vi "UHR-Fleezers Control (fpga) - avogadro 4.vi"() -> ()   [LabVIEW 2014]
doc: "UHR-Fleezers Instrument Control Code (fpga)"
uses:
  <vilib>/Platform/TimedLoop/XDataNode/timing_clust.ctl
  <vilib>/Platform/TimedLoop/XDataNode/nitl_modes.ctl
  <vilib>/Platform/TimedLoop/XDataNode/wakeup.ctl
  <vilib>/rvi/Emulation/niFpgaGetClockAttributes.vi
  <vilib>/rvi/Emulation/niFpgaSctlEmulationGetInTimedLoop.vi
  <vilib>/rvi/Emulation/niFpgaEmulationReportErrorSimple.vi
  <vilib>/rvi/Emulation/niFpgaProcessEmulError.vi
  <vilib>/rvi/eio/common/nirviEmuTemplateMethod_errors.vi
  <vilib>/rvi/Emulation/niFpgaEmulationIsFPGAContextNoSignature.vi
  <vilib>/rvi/errors/niFpgaSetErrorForExecOnDevCompSimple.vi
  <vilib>/rvi/eio/common/nirviEmuReportErrorAndStop.vi
  <vilib>/rvi/DataTransferAndStorage/Container/Common/niFpgaContainerGetUniqueNameForEmu.vi
  <vilib>/rvi/FIFO/Fifo_Resource/nirvififoEmulationSetSize.vi
  <vilib>/rvi/FIFO/Fifo_Resource/nirviFifoEmulationQueueMgr.vi
  <instcachedir>/0/nirviFifoEmulationQueueMgr_E5CAEC123FF24DC58D834DCA3CDAA9B5.lvgen/nirviFifoEmulationQueueMgr_E5CAEC123FF24DC58D834DCA3CDAA9B5_001.vi
  <vilib>/Utility/error.llb/Clear Errors.vi
  <vilib>/rvi/FIFO/Fifo_Resource/nirvififoEmulationCreateLock.vi
  <vilib>/rvi/FIFO/Fifo_Resource/nirvififoEmulationObtainLock.vi
  <vilib>/rvi/FIFO/Fifo_Resource/nirvififoEmulationReleaseLock.vi
  <vilib>/rvi/occurrence/nirviWaitOnOccurrenceBase.vi
  <vilib>/rvi/errors/nirviReportUnexpectedCaseInternalError.vi
  <vilib>/rvi/errors/nirviReportUnexpectedCaseInternalError (U32).vi
  <vilib>/rvi/DataTransferAndStorage/Container/Common/niFpgaContainerExecOnDevCompGetState.vi
  <vilib>/rvi/FIFO/Fifo_Resource/nirvififoEmulationDetermineInputValidOut.vi
  <vilib>/rvi/interface/RandomDataEmulation/niFpgaRandomDataHandleErrors.vi
  <vilib>/rvi/Emulation/niFpgaCriticalErrorInLSC.vi
  <vilib>/rvi/Memory/Memory_Emulation/niFpgaMemoryEmulationCacheClearOnFirstRun.vi
  <vilib>/rvi/Memory/Memory_Emulation/nirvimemoryEmulationManagerCache_MakeExclusive.vi
  <vilib>/rvi/Memory/Memory_Emulation/niFpgaMemoryEmulationValidateCache.vi
  <vilib>/rvi/Memory/Memory_Emulation/nirvimemoryEmulationManagerCache_InsertValue.vi
  <vilib>/rvi/Memory/Memory_Emulation/nirvimemoryEmulationManagerCache_ReleaseExclusive.vi
  <vilib>/rvi/Memory/Memory_Emulation/nirvimemoryEmulationManagerCache_GetValue.vi
  <vilib>/rvi/Memory/Memory_Emulation/nirvimemoryEmulationManagerCache_SetValue.vi
  <vilib>/rvi/Emulation/niFpgaSctlEmulationResourceMgr.vi
  <vilib>/eio/EIONode/EIONode.xnode
  <vilib>/eio/EIOMethodNode/EIOMethodNode.xnode
  <vilib>/Platform/TimedLoop/XDataNode/XDataNode.xnode
  <vilib>/rvi/DataTransferAndStorage/Container/XNode/niFpgaContainer.xnode
  <vilib>/rvi/FIFO/Fifo_Resource/nirvififoEmulationRead.vi
  <vilib>/rvi/FIFO/Fifo_Resource/niFpgaFifoEmulationRefIn.vi
  <vilib>/rvi/interface/RandomDataEmulation/nirviRandomDataFpgaReadWriteTemplate.vi
  <vilib>/rvi/FIFO/Fifo_Resource/nirvififoEmulationWrite.vi
  <vilib>/rvi/Memory/Memory_Emulation/niFpgaMemoryEmulationRefIn.vi
  <vilib>/addons/control/pid/fpga.llb/XNode/niFpgaPID.xnode
  <vilib>/Platform/TimedLoop/XDataNode/XDNodeRunTimeDep.lvlib
panel:
  in  "BD 1 Delay (ticks)":u8
  out "lifetime (ticks)":u16
  in  "Lifetime to FIFO":bool
  in  "Tab Control":T1(tab)=enum."MCL trap control"
  in  "Set 3":bool
  in  "Set 2":bool=TRUE
  in  "Set 1":bool=TRUE
  in  "Trap Pos to FIFO":bool
  in  "N of AI1 Int Acq Sets":i16=2 min=1 max=3 step=1
  out "AI Late Counter":u8
  in  "ai count":u16=400
  in  "+ phase":bool
  in  "Phase count adjustment":i16
  out "Relative phase":i16
  in  "AI to FIFO":bool
  out "BD1 Frequency Out 1":u64
  out "BD1 Frequency Out 2":u64
  out "Trap Pos FIFO Timeout":u16
  out "Trap AI FIFO Timeout":u16
  in  "Trap FIFO Set Timeout":i32
  in  "Tab Control 2":T2(tab)
  in  "Multiple trap 3 position offset \nfile":bool
  in  "Piezo offset Y points":u64
  in  "Piezo offset X points":u64
  in  "Piezo offset Xmin":u64
  in  "Piezo Offset Ymin":u64
  in  "Piezo Offset Increment":u64
  out "BD1 amplitude 1 out":u16
  out "BD1 amplitude 2 out":u16
  in  "FB output range":cluster{"output low":i16, "output high":i16}={"output low"=0, "output high"=3000}
  in  "FB Gains":T3={"proportional gain (Kc)"=10, "integral gain (Kc*Ts/Ti)"=5, "derivative gain (Kc*Td/Ts)"=0}
  in  "RF synth green feedback max":i16=4000
  in  "RD":bool=TRUE
  in  "Swap F1 and F2":bool
  in  "Cont. Scan":bool
  in  "Abort scan":bool
  in  "Cycles per step":u64
  in  "Scan BD":bool
  in  "Number of scans":u16
  in  "Scan steps":u64
  in  "Scan freq.  increment":i64
  out "Scanning":bool
  in  "Start scan":bool
  in  "OSK Bd 1":bool
  in  "Reset Bd 1":bool
  in  "PMODE":bool=TRUE
  in  "Number Interlace Cycles":u8=2 min=1 max=3
  in  "Interlace Off Parameters":u8=1 min=1 max=3
  in  "Interlace ON/OFF":bool
  out "DIO Relative phase":i16
  in  "Phase count adjustment (DIO)":i16
  in  "+ phase (DIO)":bool
  out "DIO Late Counter":u8
  in  "DIO count 1 (ticks)":u16=400
  in  "DIO count 2 (ticks)":u16=400
  in  "DIO count 3 (ticks)":u16=400
  out "AI2 Y Sum Set 2":i16
  out "AI2 Y Sum Set 1":i16
  in  "FB Setpoint Set 1":i16 min=0 step=1
  in  "FB Reset Set 1":bool
  in  "FB On/Off Set 1":bool
  in  "FB Reset Set 2":bool
  in  "FB On/Off Set 2":bool
  in  "FB Setpoint Set 2":i16 min=0 step=1
  out "Scan I":u64
  in  "Amp switch delay":u8=5
  in  "RF synth bd controls green":bool
  in  "Phase Trap 2":fxp<+,14,14>
  in  "Phase Trap 1":fxp<+,14,14>
  in  "Phase offset method":u8
  in  "BD 2 Amplitude 1":u16
  in  "BD 1 Amplitude 1":u16
  in  "BD 2 Frequency 1":u64
  in  "BD 1 Frequency 1":u64
  in  "BD 2 Amplitude 2":u16
  in  "BD 1 Amplitude 2":u16
  in  "BD 2 Frequency 2":u64
  in  "BD 1 Frequency 2":u64
  in  "BD 2 Amplitude 3":u16
  in  "BD 1 Amplitude 3":u16
  in  "BD 2 Frequency 3":u64
  in  "BD 1 Frequency 3":u64
  in  "BD 2 Delay (Ticks)":u8 caption="Count(Ticks)"
  in  "Next trap write delay (ticks)":u8 caption="Count(Ticks)"
  out "Random phase generated":fxp<+,14,14>
  in  "RF phase reset before cycles":bool
  in  "Trap 1 osc enable":bool
  in  "N trap osc periods":i16
  in  "Trap osc period (pts)":i16
  in  "Osc traps":bool
  in  "Initiate trap osc":bool
  in  "Ready Write":bool
  in  "Data":i64
  in  "Address 2":u32
  in  "Osc trap cont.":bool
  in  "Trap 2 osc enable":bool
  out "Piezo X out":i16
  out "Piezo Y out":i16
  in  "Piezo Trap ON/Off (AO3)":i16
  in  "Piezo Trap X (AO5)":i16
  in  "Piezo Trap Y (AO4)":i16
  in  "FB Min frequency":u64
  in  "FB Max Frequency":u64
  in  "Dynamic Force FB (Ronen)":bool
  in  "Trap pos. FB Range":T4={"FB2 output low"=-1.0, "FB2 output high"=0.999969482421875}
  in  "Trap Pos. FB Gains":T5={"proportional gain (Kc)"=0.999969482421875, "integral gain (Kc*Ts/Ti)"=0.999969482421875, "derivative gain (Kc*Td/Ts)"=0.0}
  in  "B factor":fxp<+/-,32,16>
  in  "Negate Diff?":bool
  in  "Diff FB Measurement?":bool
  in  "FB Trig Integrate":u32=1
  out "TTrig?":bool
  in  "TTrig Negate Pos":bool=TRUE
  out "Trap Pos FB Int Signal":fxp<+/-,24,9> format="%.18g"
  out "Trap Pos FB Int-Norm Signal":fxp<+/-,16,1> format="%.16g"
  in  "FPGA TTrig Thresh":i64
  in  "FPGA Trap Trig":bool
  out "Trap Pos FB Action":i64
  in  "Trap Pos. FB Offset Factor":i64
  in  "Trap Pos. FB Mult Factor":i64=2
  in  "Trap Pos. FB Reset":bool
  in  "Trap Pos FB Monitor T1 or T2":bool
  in  "AI1 X Scale":u16
  in  "Trap Pos FB Int Count":u16=100
  in  "Trap Pos FB Negate Action":bool
  out "AI1 X Set 2":fxp<+/-,16,1>
  out "AI1 X Set 1":fxp<+/-,16,1>
  in  "Trap Pos. FB SP":fxp<+/-,16,1>
  in  "Force feedback":bool
  out "TTrig Sig":i64
  out "TTrig Fin Thresh":i64
  in  "ScanTrap 3 or Fl-laser":bool
  in  "1D or 2D Scan?":bool
  in  "Abort scan (MCL)":bool
  in  "MCL Scan Axis":bool
  in  "Cont. Scan (MCL)":bool
  out "Scan I (MCL)":u64
  in  "Number of scans (MCL)":u16
  out "Scanning MCL":bool
  in  "Scan steps (MCL)":u64
  in  "Cycles per step (MCL)":u64
  in  "Scan freq.  increment (MCL)":i16
  in  "Start scan (MCL)":bool
  in  "AO2 (X)":i16
  in  "AO1 (Y)":i16
  out "MCL Late Counter":u8
  in  "MCL count":u32=800
  out "MCL Relative Phase":i16
  in  "Phase count adjustment (MCL)":i16
  in  "+ phase (MCL)":bool
  in  "Lifetime events to read blue":u16=100
  in  "Lifetime read blue fifo":bool
  out "lifetime events in fifo":u16
  out "APD2 int gate":bool
  out "APD3 out state":bool
  in  "APD Gate Operating Mode":u8 max=2 step=1
  in  "Invert APD Gate":bool
  in  "APD Gate OFF Count":u16=100
  in  "APD Gate ON Count":u16=300
  out "APD 1 Gate Late Counter":u8
  out "APD 1 Gate Relative Phase":i16
  in  "Phase count adjustment (APD 1 Gate)":i16
  in  "+ phase (APD 1 Gate)":bool
  out "APD 2 Counts 0":u32
  out "APD 2 Counts 1":u32
  out "APD 1 Counts 0":u32
  out "APD 1 Counts 1":u32
  out "APD1 out state":bool
  in  "APD AO scale factor":i16=1
  in  "APD to FIFO":bool
  in  "APD Acq Rate Count":u32=20000000
  out "APD Acq Late Counter":u8
  out "APD Acq Relative Phase":i16
  in  "Phase Count Adjustment (APD Acq)":i16
  in  "+ phase (APD Acq)":bool
  in  "Phase count adjustment (APD 2 Gate)":i16
  out "APD 2 Gate Late Counter":u8
  out "APD 2 Gate Relative Phase":i16
  in  "+ phase (APD 2 Gate)":bool
  out "APD2 out state":bool
  out "APD 3 Counts 0":u32
  out "APD 3 Counts 1":u32
  out "APD 3 Gate Late Counter":u8
  in  "Phase count adjustment (APD 3 Gate)":i16
  out "APD 3 Gate Relative Phase":i16
  in  "+ phase (APD 3 Gate)":bool
  out "APD1 int gate":bool
  out "APD3 int gate":bool
  in  "Lifetime timeout APD1":u16=200
  in  "D3 2":i16
  in  "I3 2":i16=5
  in  "P3 2":i16=10
  in  "Green FB Setpoint 2":i16=250 min=0 step=1
  in  "Green FB Reset 2":bool
  in  "ALEX ON":bool
  out "ALEX green ON":bool=TRUE
  in  "ALEX green on count":i16=1
  in  "D3":i16
  in  "I3":i16=5
  in  "P3":i16=10
  in  "Green Filter Flipper":bool
  in  "Green FB Count":u16=1200
  out "Green Late Counter":u8
  out "Green FB Relative Phase":i16
  in  "Phase count adjustment (Green FB)":i16=10
  in  "+ phase (Green FB)":bool
  out "Green FB Sum":i16
  in  "Green int current ON count adj":u16=150
  in  "Current Out":u16=30000
  in  "Green FB On/Off":bool
  in  "Green FB Setpoint":i16=250 min=0 step=1
  in  "Green FB Reset":bool
  in  "Operating Mode 2":u8=2 max=2 step=1
  in  "Invert GI 2":bool
  in  "Green interlace OFF count 2":u16=900
  in  "Green interlace ON count 2":u16=300
  out "GI Late Counter 2":u8
  out "GI Relative phase 2":i16
  in  "Phase count adjustment (GI) 2":i16=20
  in  "+ phase (GI) 2":bool
  in  "Green interlace OFF count":u16=100
  out "GI Relative phase":i16
  in  "Phase count adjustment (GI)":i16
  in  "+ phase (GI)":bool
  in  "Green interlace ON count":u16=300
  out "GI Late Counter":u8
  in  "Invert GI":bool
  in  "Operating Mode":u8 max=2 step=1
  in  "ALEX red on count":i16=1
  out "ALEX red ON":bool=TRUE
  out "green FB running":bool
  in  "+ phase (RI)":bool
  out "RI Relative phase":i16
  out "RI Late Counter":u8
  in  "Red interlace ON count":u16=300
  in  "Red interlace OFF count":u16=100
  in  "Invert RI":bool
  in  "Red Laser Operating Mode":u8 max=2 step=1
  in  "Phase count adjustment (RI)":i16
  out "Red FB Intensity":i16
  in  "RI Current Out":u16=30000
  in  "Red FB On/Off":bool
  in  "D4":i16
  in  "I4":i16=5
  in  "P4":i16=10
  in  "Red FB Setpoint":i16=250 min=0 step=1
  in  "Red FB Reset":bool
  in  "RI Operating Mode 2":u8=2 max=2 step=1
  in  "Invert RI 2":bool
  in  "Phase count adjustment (BI AO)":i16=20
  in  "Blue current ON count adj (AO)":u16=150
  in  "BI Current Out":i16=30000
  in  "Blue FB On/Off":bool
  in  "D5":i16
  in  "I5":i16=5
  in  "P5":i16=10
  in  "Blue FB Setpoint":i16=250 min=0 step=1
  in  "Blue FB Reset":bool
  in  "BI Operating Mode (AO)":u8=2 max=2 step=1
  in  "Invert BI (AO)":bool
  in  "Blue OFF count (AO)":u16=900
  in  "Blue ON count (AO)":u16=300
  out "BI Late Counter (AO)":u8
  out "BI Relative phase (AO)":i16
  in  "+ phase (BI AO)":bool
  in  "Phase count adjustment (BI D)":i16
  in  "Blue Laser Operating Mode (D)":u8 max=2 step=1
  in  "Invert BI (D)":bool
  in  "Blue interlace OFF count (D)":u16=100
  in  "Blue interlace ON count (D)":u16=300
  out "Blue Late Counter (D)":u8
  out "BI Relative phase (D)":i16
  in  "+ phase (BI D)":bool
  out "Blue Intensity":i16
  # "Raster Scan AOD"
  # "1 (X)"
  # "2 (Y)"
  # "IR Intensity Feedback (RF BD 1)"
  # "FB Gains Set 1"
  # "FB output range 1"
  # "IR Intensity Feedback (RF BD 2) -\nonly when using BD 2 for green laser AOM (not trap Y)"
  # "Keep below 4096 (12 bits) to stay within range of RF board. Going over doesn't saturate, it truncates higher bits."
  # "RF phase offset control"
  # "Methods are:\n0 - Default, do nothing at all (no phase offset writes)\n1 - Manual phase adjustment\n2 - Cycle the phase adjustment using the input phase numbers as increment values for each cycle"
  # "False is usual, True is external loop method"
  # "Parameters if using the external RF switching loop"
  # "Parameters if using the usual internal RF switching method"
  # "FB Triggering Excitation Laser"
  # "Trap Pos. FB Gains"
  # "Trap Pos. FB Range"
  # "AO1 (Y)"
  # "2D"
  # "Trap 3"
  # "1D"
  # "AO2 (X)"
  # "Fl Laser"
  # "APD AO for aligning"
  # "Detection Loop"
  # "Green fluorescent laser digital gate interlacing loop"
  # "0 Forced ON\n1 Forced OFF\n2 Interlacing"
  # "ALEX settings:"
  # "Controls for usual IA ME controls green AOM"
  # "Controls for RF synth board controls green AOM"
  # "Green FB Gains"
  # "Red fluorescent laser digital gate interlacing loop"
  # "Detection Loop"
  # "0 Forced ON\n1 Forced OFF\n2 Interlacing"
  # "Analog/FB Control Loop\n(Disabled)"
  # "Digital Control Loop"
  # "Blue laser intensity reading"
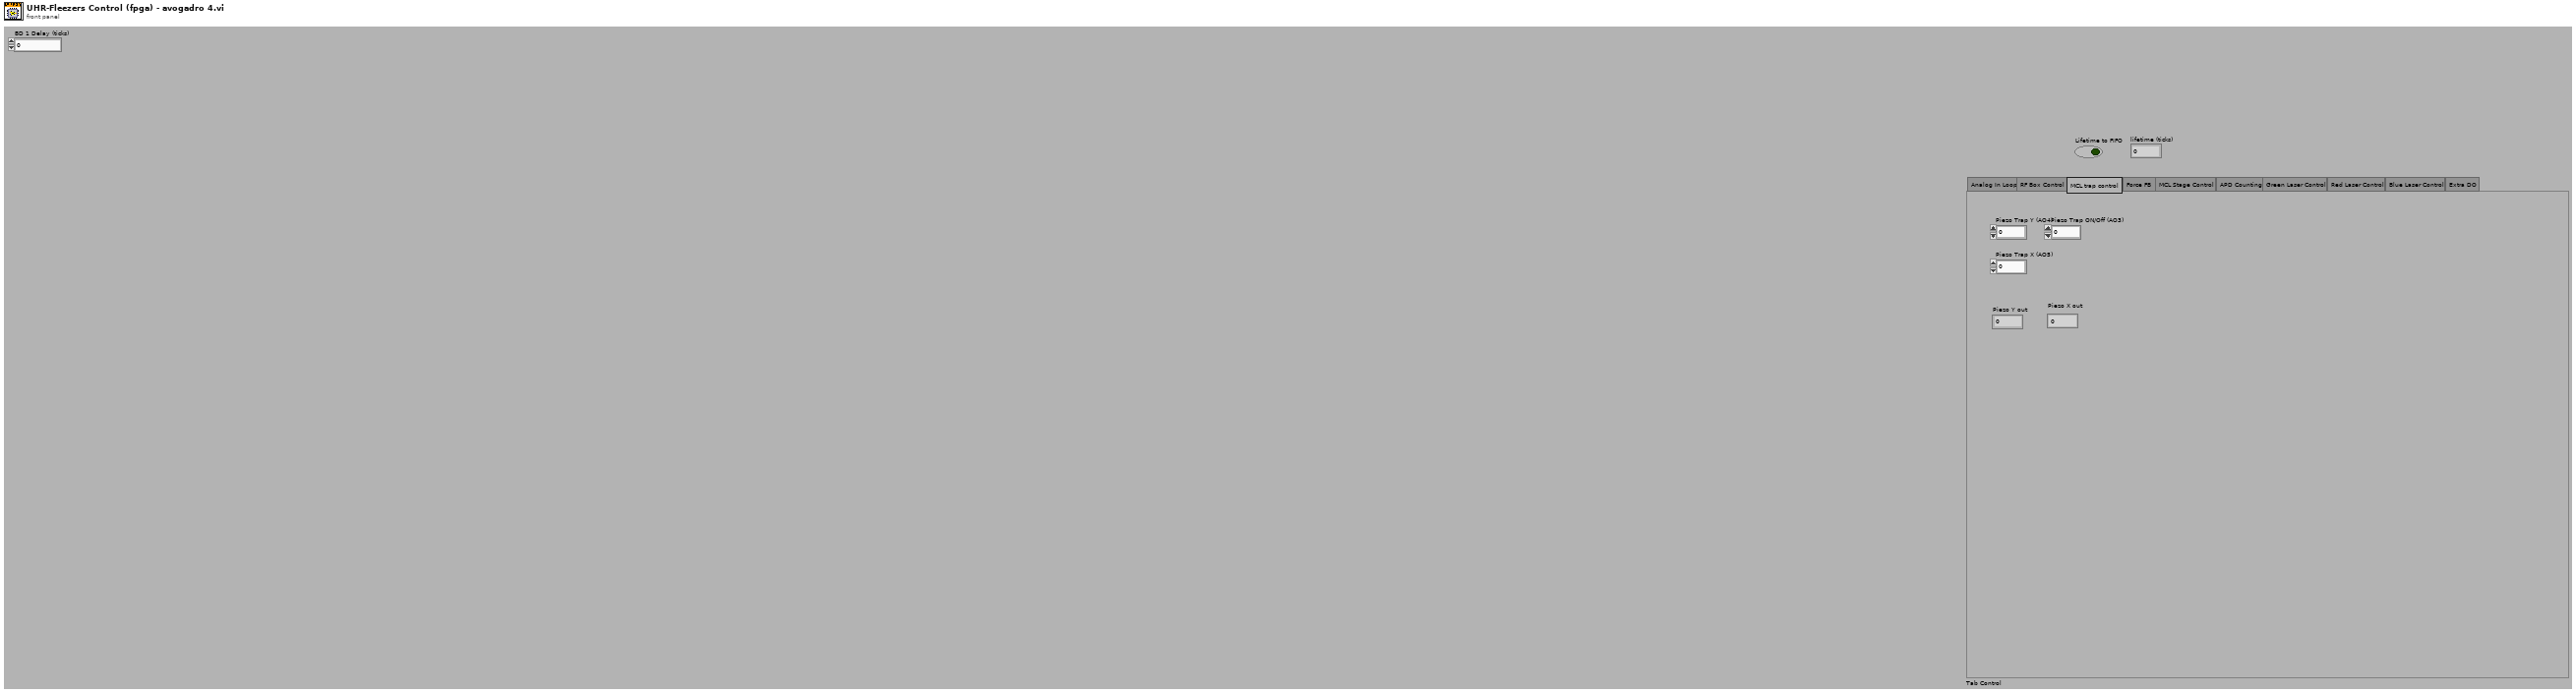
[diagram p1: front panel]
types:
  T1 = enum32{"Analog In Loop", "RF Box Control", "MCL trap control", "Force FB", "MCL Stage Control", "APD Counting", "Green Laser Control", "Red Laser Control", "Blue Laser Control", "Extra DO"}
  T2 = enum32{"Controls", "Interlacing Frequency and Amplitude Values", "Oscillate trap from memory"}
  T3 = cluster{"proportional gain (Kc)":i16, "integral gain (Kc*Ts/Ti)":i16, "derivative gain (Kc*Td/Ts)":i16}
  T4 = cluster{"FB2 output low":fxp<+/-,16,1>, "FB2 output high":fxp<+/-,16,1>}
  T5 = cluster{"proportional gain (Kc)":fxp<+/-,16,1>, "integral gain (Kc*Ts/Ti)":fxp<+/-,16,1>, "derivative gain (Kc*Td/Ts)":fxp<+/-,16,1>}
  T6 = typedef "XDNodeRunTimeDep.lvlib/timing_clust.ctl" = cluster{"Expected End [f-1]":u64, "Actual End [f-1]":u64, "Finished Late? [f-1]":bool, "Expected End [i-1]":u64, "Actual End [i-1]":u64, "Finished Late? [i-1]":bool, "Expected Start [i]":u64, "Actual Start [i]":u64, "Expected Start [f]":u64, "Actual Start [f]":u64, "Source Name":string, "Structure Name":string, "Period":i64, "Deadline":i64, "Offset":i64, "Start":i64, "Priority":i32, "Timeout":i32, "Mode":T7, "Wakeup Reason":T8, "Error":errorcluster, "Source Type":string, "Secondary Source Type":string, "Global End Time":u64, "Global Start Time":u64, "Frame Duration":u64, "Iteration Duration":u64, "Assigned CPU":i32, "I/O Scan Engine Mode":u32}
  T7 = typedef "XDNodeRunTimeDep.lvlib/nitl_modes.ctl" = enum32{"No Change", "Process missed periods, maintain original phase", "Discard missed periods, maintain original phase", "Process missed periods, ignore original phase", "Discard missed periods, ignore original phase"}
  T8 = typedef "XDNodeRunTimeDep.lvlib/wakeup.ctl" = enum32{"Normal", "Aborted", "Asynchronous wakeup", "Timing source error", "Timed loop error", "Timeout"}
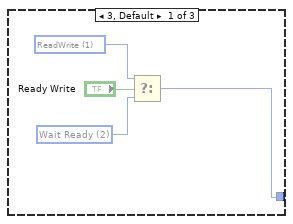
[diagram p2: hidden frame]
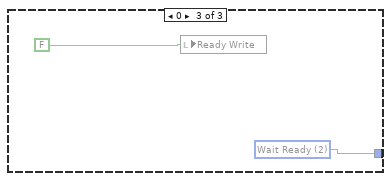
[diagram p3: hidden frame]
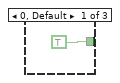
[diagram p6: hidden frame]
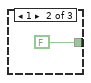
[diagram p7: hidden frame]
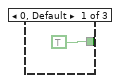
[diagram p8: hidden frame]
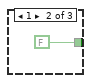
[diagram p9: hidden frame]
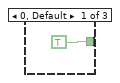
[diagram p13: hidden frame]
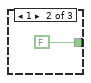
[diagram p14: hidden frame]
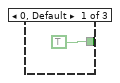
[diagram p19: hidden frame]
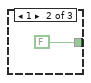
[diagram p20: hidden frame]
diagram:
  w2 = i16 0
  w6 = TRUE
  # "BD2 amp"
  # "BD1 amp"
  # "BD2 amp"
  # "BD1 amp"
  # "timing array current index"
  # "timing array"
  # "timing counter (phase adjusted here)"
  # "late counter"
  n1 = disable-structure shown="Disabled" {
    frame Disabled {
      w13 = i16 2 items=["UnSet Ready", "ReadWrite", "Wait Ready"]
      n2 = while "Handshake memory transfer for trap oscillation sin wave data" {
        shift-right: [w15] -> _
        shift-left: w13 -> [w16]
        stop <- FALSE stop-if-true
        # "Write"
        n3 = case shown="1" w16 {
          tunnel: [w19 w24 w25] -> w15
          frame 3, Default {
            w17 = i16 2 items=["UnSet Ready", "ReadWrite", "Wait Ready"]
            w18 = i16 1 items=["UnSet Ready", "ReadWrite", "Wait Ready"]
            n4 = Select(t=w18, s="Ready Write", f=w17) -> (s? t:f=w19:i16)
          }
          frame 1 {
            w24 = i16 0 items=["UnSet Ready", "ReadWrite", "Wait Ready"]
            n5 = xnode ("Memory Write")("Address"="Address 2", "Data"="Data", "Memory In"=refnum<k21> "Trap osc memory") -> ()  [unwired: 1 out]
          }
          frame 0 {
            w25 = i16 2 items=["UnSet Ready", "ReadWrite", "Wait Ready"]
            n6 = local write "Ready Write"(FALSE ("Ready Read")) -> ()
          }
        }
      }
    }
    frame Enabled {
    }
  }
  n7 = flat-sequence "FPGA initialization to do before running any of the loops" {
    tunnel: [u16 0 ("DIO count 3 (ticks)")] -> w5
    tunnel: [w34] -> _
    frame #0 {
      # "UDCLK out enable and set low"
      # "WR"
      # "BD 2"
      # "BD 1"
      # "With the RF synth board initialization now done in a separate fpga vi, now when this vi is started, board is already configured and is ready for interlacing. Just need to set WR high and enabled UDCLK as write and set to low.\nbefore setting data and address bits."
      # "Start up expansion chassis early\nto avoid delays later"
      # "Set data and address values to something safe (a correct setting) so any initial WR and udclk flipping doesn't have a chance to mess anything up. Safe would be setting an unused data entry:"
      n8 = xnode "FPGA I/O Method Node"("Enable"=TRUE) -> ("FPGA I/O Out"=w28:refnum<k21>)  [unwired: 1 in]
      n9 = xnode "FPGA I/O Method Node"("Enable"=TRUE) -> ("FPGA I/O Out"=w31:refnum<k21>)  [unwired: 1 in]
      n10 = xnode "FPGA I/O Node"("Chassis2/Mod1/AO0"=u16 0 ("Chassis2/Mod4/AO0")) -> ("Chassis2/Mod2/AI0"=w34:i16)  [unwired: 2 in, 2 out]
      n11 = xnode "FPGA I/O Node"("Connector1/DIO15"=TRUE) -> ()  [unwired: 1 in, 1 out]
      n12 = xnode "FPGA I/O Node"("I/O Item"=FALSE ("Connector1/DIO30"), "FPGA I/O In"=w28) -> ()  [unwired: 1 out]
      n13 = xnode "FPGA I/O Node"("I/O Item"=FALSE ("Connector1/DIO30"), "FPGA I/O In"=w31) -> ()  [unwired: 1 out]
      n14 = xnode "FPGA I/O Node"("Connector1/DIO0"=FALSE, "Connector1/DIO1"=FALSE, "Connector1/DIO2"=FALSE, "Connector1/DIO3"=FALSE, "Connector1/DIO4"=FALSE, "Connector1/DIO5"=FALSE, "Connector1/DIO6"=FALSE, "Connector1/DIO7"=FALSE, "Connector1/DIO8"=FALSE, "Connector1/DIO9"=FALSE, "Connector1/DIO10"=FALSE, "Connector1/DIO11"=FALSE, "Connector1/DIO12"=FALSE, "Connector1/DIO13"=FALSE, "Connector1/DIO20"=FALSE, "Connector1/DIO21"=FALSE, "Connector1/DIO22"=FALSE, "Connector1/DIO23"=FALSE, "Connector1/DIO24"=FALSE, "Connector1/DIO25"=FALSE, "Connector1/DIO26"=FALSE, "Connector1/DIO27"=FALSE, "Connector1/DIO14"=FALSE) -> ()  [unwired: 23 in, 23 out]
    }
  }
  n15 = node-c288() -> (w9:T6)  [unwired: 1 in]
  n16 = timed-loop "RF box board DIO control: control bits" {
    timing: w9 -> [_]
    timing-out: [_] -> w8
    tunnel: [w62] -> _
    tunnel: w5 -> [w62]
    stop <- FALSE stop-if-true
    n17 = xnode "FPGA I/O Node"("Connector1/DIO16"="RD", "Connector1/DIO17"="PMODE", "Connector1/DIO18"="OSK Bd 1", "Connector1/DIO19"="Reset Bd 1", "Connector0/DIO3"="Green Filter Flipper") -> ()  [unwired: 5 in, 5 out]
  }
  n18 = node-c288(w8) -> ()
  n19 = local read "AO1 (Y)"() -> (w11:i16)
  n20 = local read "AO2 (X)"() -> (w10:i16)
  n21 = disable-structure shown="Disabled" {
    disable-tunnel: w5 -> [w69 _]
    frame Disabled {
      n22 = while "APD 2 Counter" {
        tunnel: w69 -> [_]
        stop <- FALSE stop-if-true
        n23 = flat-sequence {
          frame #0 {
            n24 = xnode "FPGA I/O Method Node"("FPGA I/O In"=refnum<k21> "Connector0/DIO8" ("APD 2 DO"), "Timeout"=-1) -> ()  [unwired: 2 out]
          }
          frame #1 {
            n25 = local read "APD2 int gate"() -> (w91:bool)
            n26 = case shown="True" w91 {
              frame False {
              }
              frame True {
                n27 = local read "APD2 out state"() -> (w92:bool)
                n28 = case shown="False" w92 {
                  frame False {
                    n29 = local read "APD 2 Counts 0"() -> (w94:u32)
                    n30 = Increment(x=w94) -> (x+1=→"APD 2 Counts 0":u32)
                  }
                  frame True {
                    n31 = local read "APD 2 Counts 1"() -> (w96:u32)
                    n32 = Increment(x=w96) -> (x+1=→"APD 2 Counts 1":u32)
                  }
                }
              }
            }
          }
        }
      }
      n33 = while "APD 1 Counter" {
        tunnel: w69 -> [_]
        stop <- FALSE stop-if-true
        n34 = flat-sequence {
          frame #0 {
            n35 = xnode "FPGA I/O Method Node"("FPGA I/O In"=refnum<k21> "Connector0/DIO4" ("APD 1 DO"), "Timeout"=-1) -> ()  [unwired: 2 out]
          }
          frame #1 {
            n36 = local read "APD1 int gate"() -> (w82:bool)
            n37 = case shown="True" w82 {
              frame False {
              }
              frame True {
                n38 = local read "APD1 out state"() -> (w83:bool)
                n39 = case shown="True" w83 {
                  frame False {
                    n40 = local read "APD 1 Counts 0"() -> (w85:u32)
                    n41 = Increment(x=w85) -> (x+1=→"APD 1 Counts 0":u32)
                  }
                  frame True {
                    n42 = local read "APD 1 Counts 1"() -> (w87:u32)
                    n43 = Increment(x=w87) -> (x+1=→"APD 1 Counts 1":u32)
                  }
                }
              }
            }
          }
        }
      }
      n44 = while "APD 3 Counter" {
        tunnel: w69 -> [_]
        stop <- FALSE stop-if-true
        n45 = flat-sequence {
          frame #0 {
            n46 = xnode "FPGA I/O Method Node"("FPGA I/O In"=refnum<k21> "Connector0/DIO12" ("APD 2 DO"), "Timeout"=-1) -> ()  [unwired: 2 out]
          }
          frame #1 {
            n47 = local read "APD3 int gate"() -> (w73:bool)
            n48 = case shown="True" w73 {
              frame False {
              }
              frame True {
                n49 = local read "APD3 out state"() -> (w74:bool)
                n50 = case shown="True" w74 {
                  frame False {
                    n51 = local read "APD 3 Counts 0"() -> (w76:u32)
                    n52 = Increment(x=w76) -> (x+1=→"APD 3 Counts 0":u32)
                  }
                  frame True {
                    n53 = local read "APD 3 Counts 1"() -> (w78:u32)
                    n54 = Increment(x=w78) -> (x+1=→"APD 3 Counts 1":u32)
                  }
                }
              }
            }
          }
        }
      }
    }
    frame Enabled {
    }
  }
  n55 = To Unsigned Long Integer(number=w5) -> (unsigned 32bit integer=w7:u32)
  n56 = disable-structure shown="Disabled" {
    disable-tunnel: w5 -> [w97 _]
    frame Disabled {
      w98 = FALSE
      n57 = while "APD 1 Gating" {
        shift-right: [w204] -> _
        shift-left: w97 -> [w209]
        shift-right: [w203] -> _
        shift-left: w98 -> [w201]
        stop <- FALSE stop-if-true
        n58 = flat-sequence {
          tunnel: w209 -> [w212]
          tunnel: [w213] -> w207
          tunnel: [w212] -> w205
          tunnel: [w211] -> w202
          tunnel: w201 -> [w211]
          tunnel: [w216] -> w208
          tunnel: w207 -> [w216]
          tunnel: [w215] -> w206
          tunnel: w205 -> [w215]
          tunnel: w202 -> [w214]
          tunnel: [w234] -> w204
          tunnel: w208 -> [w248]
          tunnel: w206 -> [w245]
          tunnel: [w217] -> w203
          frame #0 {
            n59 = call "Loop Timer7"("Count(Ticks)"=w212) -> ("Tick Count(Ticks)"=w213:u16)
          }
          frame #1 {
            # "Signal maybe then sent through \na transistor before APD"
            n60 = xnode "FPGA I/O Node"("Connector0/DIO0"=w214) -> ()  [unwired: 1 in, 1 out]
            "APD1 int gate" <- w214
          }
          frame #2 {
            n61 = feedback #1(TRUE) -> (w240:bool)
            n62 = feedback-in #2(w248) -> ()
            n63 = feedback #2(w248) -> (w247:u16)
            n64 = Not(x=w240) -> (.not. x?=w237:bool)
            n65 = feedback-in #1(w237) -> ()
            n66 = Subtract(x=w248, y=w247) -> (x-y=w246:u16)
            n67 = Select(t="APD Gate ON Count", s=w237, f="APD Gate OFF Count") -> (s? t:f=w242:u16)
            n68 = Subtract(x=w246, y=w245) -> (x-y=w222:u16)
            n69 = Subtract(x=w242, y=w222) -> (x-y=w233:u16)
            n70 = Number To Boolean Array(number=w222) -> (Boolean array=w223:bool[])
            n71 = Or Array Elements(Boolean array=w223) -> (logical OR=w221:bool)
            n72 = Boolean To (0,1)(Boolean="+ phase (APD 1 Gate)") -> (0, 1=w231:i16)
            n73 = Boolean To (0,1)(Boolean=w221) -> (0, 1=w228:i16)
            n74 = Multiply(x=w231, y="Phase count adjustment (APD 1 Gate)") -> (x*y=w229:i16)
            n75 = To Unsigned Byte Integer(number=w228) -> (unsigned 8bit integer=w225:u8)
            n76 = Add(x=w233, y=w229) -> (x+y=w234:u16)
            n77 = feedback #3(i16 0) -> (w236:i16)
            n78 = Subtract(x=w236, y=w229) -> (x-y=w235:i16)
            "APD 1 Gate Relative Phase" <- w235
            n79 = feedback-in #3(w235) -> ()
            n80 = feedback #4(u8 0) -> (w226:u8)
            n81 = Add(x=w225, y=w226) -> (x+y=w224:u8)
            "APD 1 Gate Late Counter" <- w224
            n82 = feedback-in #4(w224) -> ()
            n83 = case shown="2" "APD Gate Operating Mode" {
              tunnel: [TRUE FALSE w251] -> w218
              tunnel: w240 -> [_ _ w251]
              frame 0, Default {
              }
              frame 1 {
              }
              frame 2 {
              }
            }
            n84 = Not(x=w218) -> (.not. x?=w219:bool)
            n85 = Select(t=w219, s="Invert APD Gate", f=w218) -> (s? t:f=w217:bool)
          }
        }
      }
      n86 = while "APD 2 Gating" {
        shift-right: [w153] -> _
        shift-left: w97 -> [w158]
        shift-right: [w152] -> _
        shift-left: w98 -> [w150]
        stop <- FALSE stop-if-true
        n87 = flat-sequence {
          tunnel: w158 -> [w161]
          tunnel: [w162] -> w156
          tunnel: [w161] -> w154
          tunnel: [w160] -> w151
          tunnel: w150 -> [w160]
          tunnel: [w165] -> w157
          tunnel: w156 -> [w165]
          tunnel: [w164] -> w155
          tunnel: w154 -> [w164]
          tunnel: w151 -> [w163]
          tunnel: [w187] -> w153
          tunnel: w157 -> [w197]
          tunnel: w155 -> [w195]
          tunnel: [w166] -> w152
          frame #0 {
            n88 = call "Loop Timer8"("Count(Ticks)"=w161) -> ("Tick Count(Ticks)"=w162:u16)
          }
          frame #1 {
            # "Signal maybe then sent through \na transistor before APD"
            n89 = xnode "FPGA I/O Node"("Connector0/DIO1"=w163) -> ()  [unwired: 1 in, 1 out]
            "APD2 int gate" <- w163
          }
          frame #2 {
            n90 = local read "APD Gate ON Count"() -> (w180:u16)
            n91 = local read "APD Gate OFF Count"() -> (w179:u16)
            n92 = feedback #5(TRUE) -> (w192:bool)
            n93 = feedback-in #6(w197) -> ()
            n94 = feedback #6(w197) -> (w181:u16)
            n95 = Not(x=w192) -> (.not. x?=w190:bool)
            n96 = feedback-in #5(w190) -> ()
            n97 = Subtract(x=w197, y=w181) -> (x-y=w196:u16)
            n98 = Select(t=w180, s=w190, f=w179) -> (s? t:f=w194:u16)
            n99 = Subtract(x=w196, y=w195) -> (x-y=w172:u16)
            n100 = Subtract(x=w194, y=w172) -> (x-y=w186:u16)
            n101 = Number To Boolean Array(number=w172) -> (Boolean array=w171:bool[])
            n102 = Or Array Elements(Boolean array=w171) -> (logical OR=w170:bool)
            n103 = Boolean To (0,1)(Boolean="+ phase (APD 2 Gate)") -> (0, 1=w184:i16)
            n104 = Multiply(x=w184, y="Phase count adjustment (APD 2 Gate)") -> (x*y=w182:i16)
            n105 = Boolean To (0,1)(Boolean=w170) -> (0, 1=w177:i16)
            n106 = Add(x=w186, y=w182) -> (x+y=w187:u16)
            n107 = To Unsigned Byte Integer(number=w177) -> (unsigned 8bit integer=w174:u8)
            n108 = feedback #7(i16 0) -> (w189:i16)
            n109 = Subtract(x=w189, y=w182) -> (x-y=w188:i16)
            "APD 2 Gate Relative Phase" <- w188
            n110 = feedback-in #7(w188) -> ()
            n111 = feedback #8(u8 0) -> (w175:u8)
            n112 = Add(x=w174, y=w175) -> (x+y=w173:u8)
            "APD 2 Gate Late Counter" <- w173
            n113 = feedback-in #8(w173) -> ()
            n114 = local read "APD Gate Operating Mode"() -> (w178:u8)
            n115 = case shown="2" w178 {
              tunnel: [TRUE FALSE w200] -> w167
              tunnel: w192 -> [_ _ w200]
              frame 0, Default {
              }
              frame 1 {
              }
              frame 2 {
              }
            }
            n116 = local read "Invert APD Gate"() -> (w169:bool)
            n117 = Not(x=w167) -> (.not. x?=w168:bool)
            n118 = Select(t=w168, s=w169, f=w167) -> (s? t:f=w166:bool)
          }
        }
      }
      n119 = while "APD 3 Gating" {
        shift-right: [w102] -> _
        shift-left: w97 -> [w107]
        shift-right: [w101] -> _
        shift-left: w98 -> [w99]
        stop <- FALSE stop-if-true
        n120 = flat-sequence {
          tunnel: w107 -> [w110]
          tunnel: [w111] -> w105
          tunnel: [w110] -> w103
          tunnel: [w109] -> w100
          tunnel: w99 -> [w109]
          tunnel: [w114] -> w106
          tunnel: w105 -> [w114]
          tunnel: [w113] -> w104
          tunnel: w103 -> [w113]
          tunnel: w100 -> [w112]
          tunnel: [w135] -> w102
          tunnel: w106 -> [w146]
          tunnel: w104 -> [w143]
          tunnel: [w115] -> w101
          frame #0 {
            n121 = call "Loop Timer15"("Count(Ticks)"=w110) -> ("Tick Count(Ticks)"=w111:u16)
          }
          frame #1 {
            # "Signal maybe then sent through \na transistor before APD"
            n122 = xnode "FPGA I/O Node"("Connector0/DIO2"=w112) -> ()  [unwired: 1 in, 1 out]
            "APD3 int gate" <- w112
          }
          frame #2 {
            n123 = local read "APD Gate OFF Count"() -> (w120:u16)
            n124 = local read "APD Gate ON Count"() -> (w121:u16)
            n125 = feedback #9(TRUE) -> (w140:bool)
            n126 = feedback-in #10(w146) -> ()
            n127 = feedback #10(w146) -> (w145:u16)
            n128 = Not(x=w140) -> (.not. x?=w138:bool)
            n129 = feedback-in #9(w138) -> ()
            n130 = Subtract(x=w146, y=w145) -> (x-y=w144:u16)
            n131 = Select(t=w121, s=w138, f=w120) -> (s? t:f=w142:u16)
            n132 = Subtract(x=w144, y=w143) -> (x-y=w123:u16)
            n133 = Subtract(x=w142, y=w123) -> (x-y=w134:u16)
            n134 = Number To Boolean Array(number=w123) -> (Boolean array=w124:bool[])
            n135 = Or Array Elements(Boolean array=w124) -> (logical OR=w122:bool)
            n136 = Boolean To (0,1)(Boolean=w122) -> (0, 1=w129:i16)
            n137 = Boolean To (0,1)(Boolean="+ phase (APD 3 Gate)") -> (0, 1=w132:i16)
            n138 = To Unsigned Byte Integer(number=w129) -> (unsigned 8bit integer=w126:u8)
            n139 = Multiply(x=w132, y="Phase count adjustment (APD 3 Gate)") -> (x*y=w130:i16)
            n140 = feedback #11(u8 0) -> (w127:u8)
            n141 = Add(x=w126, y=w127) -> (x+y=w125:u8)
            "APD 3 Gate Late Counter" <- w125
            n142 = feedback-in #11(w125) -> ()
            n143 = Add(x=w134, y=w130) -> (x+y=w135:u16)
            n144 = feedback #12(i16 0) -> (w137:i16)
            n145 = Subtract(x=w137, y=w130) -> (x-y=w136:i16)
            "APD 3 Gate Relative Phase" <- w136
            n146 = feedback-in #12(w136) -> ()
            n147 = local read "APD Gate Operating Mode"() -> (w119:u8)
            n148 = case shown="2" w119 {
              tunnel: [TRUE FALSE w149] -> w116
              tunnel: w140 -> [_ _ w149]
              frame 0, Default {
              }
              frame 1 {
              }
              frame 2 {
              }
            }
            n149 = local read "Invert APD Gate"() -> (w118:bool)
            n150 = Not(x=w116) -> (.not. x?=w117:bool)
            n151 = Select(t=w117, s=w118, f=w116) -> (s? t:f=w115:bool)
          }
        }
      }
    }
    frame Enabled {
    }
  }
  n152 = disable-structure shown="Disabled" {
    disable-tunnel: w5 -> [w252 _]
    frame Disabled {
      n153 = while "Excitation laser intensity feedback measurement (all lasers)" {
        shift-right: [w253] -> _
        shift-left: w252 -> [w258]
        stop <- FALSE stop-if-true
        n154 = flat-sequence {
          tunnel: w258 -> [w260]
          tunnel: [w261] -> w256
          tunnel: [w260] -> w254
          tunnel: [w267] -> w257
          tunnel: w256 -> [w267]
          tunnel: [w266] -> w255
          tunnel: w254 -> [w266]
          tunnel: [w279] -> w253
          tunnel: w257 -> [w290]
          tunnel: w255 -> [w287]
          frame #0 {
            n155 = call "Loop Timer9"("Count(Ticks)"=w260) -> ("Tick Count(Ticks)"=w261:u16)
          }
          frame #1 {
            # "Design note:\n\nAll lasers need to be measured at the same \ntime because the AI expansion module\ncannot independently time the measurements\nwithin our requirements: there is dead time.\n\nThis probably wouldn't be an issue with the built\nin AI on the fpga board itself."
            n156 = xnode "FPGA I/O Node"("Connector1/DIO35"=TRUE) -> ("Chassis2/Mod1/AI2"=→"Blue Intensity", "Chassis2/Mod1/AI1"=→"Red FB Intensity", "Chassis2/Mod1/AI0"=→"Green FB Sum")  [unwired: 4 in, 4 out]
          }
          frame #2 {
            n157 = feedback-in #13(w290) -> ()
            n158 = feedback #13(w290) -> (w289:u16)
            n159 = Subtract(x=w290, y=w289) -> (x-y=w288:u16)
            n160 = xnode "FPGA I/O Node"("Connector1/DIO35"=FALSE) -> ()  [unwired: 1 in, 1 out]
            n161 = Subtract(x=w288, y=w287) -> (x-y=w269:u16)
            n162 = Subtract(x="Green FB Count", y=w269) -> (x-y=w283:u16)
            n163 = Number To Boolean Array(number=w269) -> (Boolean array=w270:bool[])
            n164 = Or Array Elements(Boolean array=w270) -> (logical OR=w268:bool)
            n165 = Boolean To (0,1)(Boolean="+ phase (Green FB)") -> (0, 1=w281:i16)
            n166 = Boolean To (0,1)(Boolean=w268) -> (0, 1=w275:i16)
            n167 = Multiply(x=w281, y="Phase count adjustment (Green FB)") -> (x*y=w276:i16)
            n168 = Add(x=w283, y=w276) -> (x+y=w279:u16)
            n169 = To Unsigned Byte Integer(number=w275) -> (unsigned 8bit integer=w272:u8)
            n170 = feedback #14(i16 0) -> (w278:i16)
            n171 = Subtract(x=w278, y=w276) -> (x-y=w277:i16)
            "Green FB Relative Phase" <- w277
            n172 = feedback-in #14(w277) -> ()
            n173 = feedback #15(u8 0) -> (w273:u8)
            n174 = Add(x=w272, y=w273) -> (x+y=w271:u8)
            "Green Late Counter" <- w271
            n175 = feedback-in #15(w271) -> ()
          }
        }
      }
    }
    frame Enabled {
    }
  }
  n176 = disable-structure shown="Disabled" {
    disable-tunnel: w5 -> [w291 _]
    frame Disabled {
      w293 = FALSE
      n177 = while "532 nm green fluorescent laser interlacing (DO to IA 532 nm AOM ME amp)." {
        shift-right: [w465] -> _
        shift-left: w291 -> [w470]
        shift-right: [w464] -> _
        shift-left: w293 -> [w462]
        stop <- FALSE stop-if-true
        n178 = flat-sequence {
          tunnel: w470 -> [w473]
          tunnel: [w474] -> w468
          tunnel: [w473] -> w466
          tunnel: [w472] -> w463
          tunnel: w462 -> [w472]
          tunnel: [w477] -> w469
          tunnel: w468 -> [w477]
          tunnel: [w476] -> w467
          tunnel: w466 -> [w476]
          tunnel: w463 -> [w475]
          tunnel: [w486] -> w465
          tunnel: w469 -> [w506]
          tunnel: w467 -> [w503]
          tunnel: [w495] -> w464
          frame #0 {
            n179 = call "Loop Timer4"("Count(Ticks)"=w473) -> ("Tick Count(Ticks)"=w474:u16)
          }
          frame #1 {
            # "Then to PRL 440 amp\nOR to RF synth board FSK in"
            n180 = xnode "FPGA I/O Node"("Connector1/DIO39"=w475) -> ()  [unwired: 1 in, 1 out]
          }
          frame #2 {
            n181 = feedback-in #16(w506) -> ()
            n182 = feedback #16(w506) -> (w505:u16)
            n183 = Subtract(x=w506, y=w505) -> (x-y=w504:u16)
            n184 = Subtract(x=w504, y=w503) -> (x-y=w479:u16)
            n185 = Number To Boolean Array(number=w479) -> (Boolean array=w480:bool[])
            n186 = Or Array Elements(Boolean array=w480) -> (logical OR=w478:bool)
            n187 = Boolean To (0,1)(Boolean="+ phase (GI)") -> (0, 1=w491:i16)
            n188 = Multiply(x=w491, y="Phase count adjustment (GI)") -> (x*y=w488:i16)
            n189 = Boolean To (0,1)(Boolean=w478) -> (0, 1=w485:i16)
            n190 = To Unsigned Byte Integer(number=w485) -> (unsigned 8bit integer=w482:u8)
            n191 = feedback #17(i16 0) -> (w489:i16)
            n192 = feedback #18(u8 0) -> (w483:u8)
            n193 = Add(x=w482, y=w483) -> (x+y=w481:u8)
            "GI Late Counter" <- w481
            n194 = feedback-in #18(w481) -> ()
            n195 = Subtract(x=w489, y=w488) -> (x-y=w487:i16)
            "GI Relative phase" <- w487
            n196 = feedback-in #17(w487) -> ()
            n197 = feedback #19(TRUE) -> (w498:bool)
            n198 = case shown="2" "Operating Mode" {
              tunnel: [TRUE FALSE w512] -> w495
              tunnel: w498 -> [_ _ w509]
              frame 0, Default {
              }
              frame 1 {
              }
              frame 2 {
                n199 = Not(x=w509) -> (.not. x?=w511:bool)
                n200 = Select(t=w511, s="Invert GI", f=w509) -> (s? t:f=w512:bool)
              }
            }
            n201 = Not(x=w498) -> (.not. x?=w494:bool)
            n202 = Select(t="Green interlace ON count", s=w494, f="Green interlace OFF count") -> (s? t:f=w500:u16)
            n203 = Subtract(x=w500, y=w479) -> (x-y=w492:u16)
            n204 = Add(x=w492, y=w488) -> (x+y=w486:u16)
            n205 = feedback-in #19(w494) -> ()
          }
        }
      }
      n206 = while "633 nm red  fluorescent laser interlacing (DO to IA 633 nm AOM ME amp)." {
        shift-right: [w414] -> _
        shift-left: w291 -> [w419]
        shift-right: [w413] -> _
        shift-left: w293 -> [w411]
        stop <- FALSE stop-if-true
        n207 = flat-sequence {
          tunnel: w419 -> [w422]
          tunnel: [w423] -> w417
          tunnel: [w422] -> w415
          tunnel: [w421] -> w412
          tunnel: w411 -> [w421]
          tunnel: [w426] -> w418
          tunnel: w417 -> [w426]
          tunnel: [w425] -> w416
          tunnel: w415 -> [w425]
          tunnel: w412 -> [w424]
          tunnel: [w435] -> w414
          tunnel: w418 -> [w455]
          tunnel: w416 -> [w452]
          tunnel: [w444] -> w413
          frame #0 {
            n208 = call "Loop Timer11"("Count(Ticks)"=w422) -> ("Tick Count(Ticks)"=w423:u16)
          }
          frame #1 {
            # "Then to PRL 440 amp"
            n209 = xnode "FPGA I/O Node"("Connector1/DIO32"=w424) -> ()  [unwired: 1 in, 1 out]
          }
          frame #2 {
            n210 = feedback-in #20(w455) -> ()
            n211 = feedback #20(w455) -> (w454:u16)
            n212 = Subtract(x=w455, y=w454) -> (x-y=w453:u16)
            n213 = Subtract(x=w453, y=w452) -> (x-y=w428:u16)
            n214 = Number To Boolean Array(number=w428) -> (Boolean array=w429:bool[])
            n215 = Or Array Elements(Boolean array=w429) -> (logical OR=w427:bool)
            n216 = Boolean To (0,1)(Boolean="+ phase (RI)") -> (0, 1=w440:i16)
            n217 = Multiply(x=w440, y="Phase count adjustment (RI)") -> (x*y=w437:i16)
            n218 = Boolean To (0,1)(Boolean=w427) -> (0, 1=w434:i16)
            n219 = To Unsigned Byte Integer(number=w434) -> (unsigned 8bit integer=w431:u8)
            n220 = feedback #21(i16 0) -> (w438:i16)
            n221 = feedback #22(u8 0) -> (w432:u8)
            n222 = Add(x=w431, y=w432) -> (x+y=w430:u8)
            "RI Late Counter" <- w430
            n223 = feedback-in #22(w430) -> ()
            n224 = Subtract(x=w438, y=w437) -> (x-y=w436:i16)
            "RI Relative phase" <- w436
            n225 = feedback-in #21(w436) -> ()
            n226 = feedback #23(TRUE) -> (w447:bool)
            n227 = case shown="2" "Red Laser Operating Mode" {
              tunnel: [TRUE FALSE w461] -> w444
              tunnel: w447 -> [_ _ w458]
              frame 0, Default {
              }
              frame 1 {
              }
              frame 2 {
                n228 = Not(x=w458) -> (.not. x?=w460:bool)
                n229 = Select(t=w460, s="Invert RI", f=w458) -> (s? t:f=w461:bool)
              }
            }
            n230 = Not(x=w447) -> (.not. x?=w443:bool)
            n231 = Select(t="Red interlace ON count", s=w443, f="Red interlace OFF count") -> (s? t:f=w449:u16)
            n232 = Subtract(x=w449, y=w428) -> (x-y=w441:u16)
            n233 = Add(x=w441, y=w437) -> (x+y=w435:u16)
            n234 = feedback-in #23(w443) -> ()
          }
        }
      }
      n235 = while "473 nm blue  fluorescent laser interlacing (DO to blue laser digital control input)." {
        shift-right: [w310] -> _
        shift-left: w291 -> [w313]
        shift-right: [w309] -> _
        shift-left: w293 -> [w307]
        shift-right: [w302] -> _
        shift-left: _ -> [w301]
        shift-right: [w294] -> _
        shift-left: u16 0 -> [w297]
        stop <- FALSE stop-if-true
        n236 = flat-sequence {
          tunnel: w313 -> [w318]
          tunnel: [w319] -> w312
          tunnel: [w318] -> w311
          tunnel: [w317] -> w308
          tunnel: w307 -> [w317]
          tunnel: w301 -> [w316]
          tunnel: [w316] -> w300
          tunnel: [w315] -> w298
          tunnel: w297 -> [w315]
          tunnel: [w324] -> w306
          tunnel: w312 -> [w324]
          tunnel: [w323] -> w305
          tunnel: w311 -> [w323]
          tunnel: w308 -> [w322]
          tunnel: w300 -> [w321]
          tunnel: [w321] -> w299
          tunnel: w298 -> [w320]
          tunnel: [w320] -> w296
          tunnel: [w329] -> w304
          tunnel: [w328] -> w303
          tunnel: w305 -> [w328]
          tunnel: w306 -> [w329]
          tunnel: w299 -> [w327]
          tunnel: w296 -> [w326]
          tunnel: [w325] -> w295
          tunnel: [w386] -> w310
          tunnel: w304 -> [w404]
          tunnel: w303 -> [w401]
          tunnel: [w374] -> w309
          tunnel: [w372] -> w302
          tunnel: w295 -> [w369]
          tunnel: [w370] -> w294
          frame #0 {
            n237 = call "Loop Timer14"("Count(Ticks)"=w318) -> ("Tick Count(Ticks)"=w319:u16)
          }
          frame #1 {
            n238 = xnode "FPGA I/O Node"("Connector1/DIO28"=w322) -> ()  [unwired: 1 in, 1 out]
          }
          frame #2 {
            n239 = case shown="True" w327 {
              tunnel: w326 -> [w330 w332]
              tunnel: [w330 w331] -> w325
              frame False {
              }
              frame True {
                n240 = flat-sequence {
                  tunnel: [w338] -> w335
                  tunnel: [w337] -> w334
                  tunnel: [w336] -> w333
                  tunnel: w332 -> [w336]
                  tunnel: w335 -> [w355]
                  tunnel: w334 -> [w352]
                  tunnel: w333 -> [w354]
                  tunnel: [w353] -> w331
                  frame #0 {
                    # "5 ns timing resolution"
                    n241 = node-c288() -> (w341:T6)  [unwired: 1 in]
                    n242 = timed-loop {
                      timing: w341 -> [_]
                      timing-out: [_] -> w340
                      tunnel: "Lifetime timeout APD1" -> [w347]
                      tunnel: [w342] -> w337
                      tunnel: [w343] -> w338
                      i -> [w344]
                      stop <- w346 stop-if-true
                      n243 = xnode "FPGA I/O Node"() -> ("Connector0/DIO5"=w345:bool)  [unwired: 1 in, 1 out]
                      n244 = To Unsigned Word Integer(number=w344) -> (unsigned 16bit integer=w342:u16)
                      n245 = Equal?(x=w347, y=w342) -> (x = y?=w343:bool)
                      n246 = Or(x=w345, y=w343) -> (x .or. y?=w346:bool)
                    }
                    n247 = node-c288(w340) -> ()
                  }
                  frame #1 {
                    n248 = Not(x=w355) -> (.not. x?=w356:bool)
                    n249 = case shown="True" w356 {
                      tunnel: w352 -> [_ w358]
                      tunnel: w354 -> [w357 w360]
                      tunnel: [w357 w359] -> w353
                      frame False {
                        # "timed out, do nothing"
                      }
                      frame True {
                        # "photon detected,record time"
                        n250 = case shown="True" "Lifetime to FIFO" {
                          tunnel: w358 -> [_ w366]
                          tunnel: w360 -> [w362 w364]
                          tunnel: [w362 w363] -> w359
                          frame False {
                            # "don't record time\n(can't if doing force feedback)"
                          }
                          frame True {
                            # "number of events in fifo"
                            n251 = xnode ("FIFO Method Node")("Element"=w366, "Timeout"=0) -> ()  [unwired: 1 in, 2 out]
                            n252 = Increment(x=w364) -> (x+1=w363:u16)
                          }
                        }
                        "lifetime (ticks)" <- w358
                      }
                    }
                  }
                }
              }
            }
          }
          frame #3 {
            # "Reading fifo is tricky here since\nunknown # of events"
            # "For lifetime measurement:\nInterlacing and pulse falling"
            n253 = feedback-in #24(w404) -> ()
            n254 = feedback #24(w404) -> (w403:u16)
            n255 = Subtract(x=w404, y=w403) -> (x-y=w402:u16)
            n256 = Subtract(x=w402, y=w401) -> (x-y=w379:u16)
            n257 = Number To Boolean Array(number=w379) -> (Boolean array=w380:bool[])
            n258 = Or Array Elements(Boolean array=w380) -> (logical OR=w378:bool)
            n259 = Boolean To (0,1)(Boolean="+ phase (BI D)") -> (0, 1=w391:i16)
            n260 = Multiply(x=w391, y="Phase count adjustment (BI D)") -> (x*y=w388:i16)
            n261 = Boolean To (0,1)(Boolean=w378) -> (0, 1=w385:i16)
            n262 = To Unsigned Byte Integer(number=w385) -> (unsigned 8bit integer=w382:u8)
            n263 = feedback #25(i16 0) -> (w389:i16)
            n264 = feedback #26(u8 0) -> (w383:u8)
            n265 = Add(x=w382, y=w383) -> (x+y=w381:u8)
            "Blue Late Counter (D)" <- w381
            n266 = feedback-in #26(w381) -> ()
            n267 = Subtract(x=w389, y=w388) -> (x-y=w387:i16)
            "BI Relative phase (D)" <- w387
            n268 = feedback-in #25(w387) -> ()
            n269 = feedback #27(TRUE) -> (w396:bool)
            n270 = case shown="2" "Blue Laser Operating Mode (D)" {
              tunnel: [TRUE FALSE w410] -> w374
              tunnel: w396 -> [_ _ w407]
              frame 0, Default {
              }
              frame 1 {
              }
              frame 2 {
                n271 = Not(x=w407) -> (.not. x?=w409:bool)
                n272 = Select(t=w409, s="Invert BI (D)", f=w407) -> (s? t:f=w410:bool)
              }
            }
            n273 = Subtract(x=w369, y="Lifetime events to read blue") -> (x-y=w367:u16)
            n274 = Not(x=w396) -> (.not. x?=w394:bool)
            n275 = Select(t="Blue interlace ON count (D)", s=w394, f="Blue interlace OFF count (D)") -> (s? t:f=w398:u16)
            n276 = Subtract(x=w398, y=w379) -> (x-y=w392:u16)
            n277 = Add(x=w392, y=w388) -> (x+y=w386:u16)
            n278 = feedback-in #27(w394) -> ()
            n279 = Select(t=w367, s="Lifetime read blue fifo", f=w369) -> (s? t:f=w370:u16)
            "lifetime events in fifo" <- w370
            n280 = Equal?(x="Blue Laser Operating Mode (D)", y=u8 2) -> (x = y?=w375:bool)
            n281 = Not(x=w374) -> (.not. x?=w373:bool)
            n282 = And(x=w373, y=w375) -> (x .and. y?=w372:bool)
          }
        }
      }
    }
    frame Enabled {
    }
  }
  n283 = disable-structure shown="Disabled" {
    disable-tunnel: w5 -> [w513 _]
    frame Disabled {
      w514 = u16 0
      n284 = while "Green and red fluorescent laser interlacing (Current AO to IA 532 nm AOM ME amp)." {
        shift-right: [w594] -> _
        shift-left: w513 -> [w597]
        shift-right: [w591] -> _
        shift-left: w514 -> [w589]
        shift-right: [w588] -> _
        shift-left: w514 -> [w587]
        stop <- FALSE stop-if-true
        n285 = flat-sequence {
          tunnel: w597 -> [w601]
          tunnel: [w602] -> w596
          tunnel: [w601] -> w595
          tunnel: [w600] -> w590
          tunnel: w589 -> [w600]
          tunnel: w587 -> [w599]
          tunnel: [w599] -> w586
          tunnel: [w606] -> w593
          tunnel: w596 -> [w606]
          tunnel: [w605] -> w592
          tunnel: w595 -> [w605]
          tunnel: w590 -> [w604]
          tunnel: w586 -> [w603]
          tunnel: [w634] -> w594
          tunnel: [w650] -> w591
          tunnel: w593 -> [w661]
          tunnel: w592 -> [w658]
          tunnel: [w619] -> w588
          frame #0 {
            n286 = call "Loop Timer10"("Count(Ticks)"=w601) -> ("Tick Count(Ticks)"=w602:u16)
          }
          frame #1 {
            n287 = xnode "FPGA I/O Node"("Chassis2/Mod4/AO0"=w604, "Chassis2/Mod4/AO1"=w603) -> ()  [unwired: 2 in, 2 out]
          }
          frame #2 {
            # "IF RF synth BD does green, never run FB"
            # "ALEX variable is used by APD acquisition loop\nto turn lasers ON/OFF."
            # "Design note:\n\nThese two laser controls are in the same loop\nbecause the expansion current AI cannot separately\ntime the outputs fast enough for us.  Apparently\nit is because of communication time between the\nexpansion card and the fpga.\n\nSo the two analog control signals have the same timing\nand profile, but independent amplitudes to independently\ncontrol the intensity and feedback for each laser."
            n288 = feedback #28(TRUE) -> (w616:bool)
            n289 = Not(x=w616) -> (.not. x?=w617:bool)
            n290 = feedback-in #28(w617) -> ()
            n291 = Subtract(x="Green interlace OFF count 2", y="Green int current ON count adj") -> (x-y=w643:u16)
            n292 = feedback-in #29(w661) -> ()
            n293 = feedback #29(w661) -> (w660:u16)
            n294 = Add(x="Green int current ON count adj", y="Green interlace ON count 2") -> (x+y=w644:u16)
            n295 = Subtract(x=w661, y=w660) -> (x-y=w659:u16)
            n296 = Select(t=w644, s=w617, f=w643) -> (s? t:f=w655:u16)
            n297 = Subtract(x=w659, y=w658) -> (x-y=w627:u16)
            n298 = case shown="2" "RI Operating Mode 2" {
              tunnel: [TRUE FALSE w667] -> w612
              tunnel: w616 -> [_ _ w664]
              frame 0, Default {
              }
              frame 1 {
              }
              frame 2 {
                n299 = Not(x=w664) -> (.not. x?=w666:bool)
                n300 = Select(t=w666, s="Invert RI 2", f=w664) -> (s? t:f=w667:bool)
              }
            }
            n301 = Subtract(x=w655, y=w627) -> (x-y=w638:u16)
            n302 = case shown="2" "Operating Mode 2" {
              tunnel: [TRUE FALSE w701] -> w614
              tunnel: w616 -> [_ _ w698]
              frame 0, Default {
              }
              frame 1 {
              }
              frame 2 {
                n303 = Not(x=w698) -> (.not. x?=w700:bool)
                n304 = Select(t=w700, s="Invert GI 2", f=w698) -> (s? t:f=w701:bool)
              }
            }
            n305 = Number To Boolean Array(number=w627) -> (Boolean array=w628:bool[])
            n306 = local read "ALEX red ON"() -> (w611:bool)
            n307 = Boolean To (0,1)(Boolean="+ phase (GI) 2") -> (0, 1=w640:i16)
            n308 = Or Array Elements(Boolean array=w628) -> (logical OR=w626:bool)
            n309 = local read "ALEX green ON"() -> (w613:bool)
            n310 = Boolean To (0,1)(Boolean=w626) -> (0, 1=w633:i16)
            n311 = Multiply(x=w640, y="Phase count adjustment (GI) 2") -> (x*y=w636:i16)
            n312 = local read "RF synth bd controls green"() -> (w608:bool)
            n313 = To Unsigned Byte Integer(number=w633) -> (unsigned 8bit integer=w629:u8)
            n314 = And(x=w611, y=w612) -> (x .and. y?=w610:bool)
            n315 = Add(x=w638, y=w636) -> (x+y=w634:u16)
            n316 = feedback #30(u8 0) -> (w631:u8)
            n317 = Add(x=w629, y=w631) -> (x+y=w630:u8)
            "GI Late Counter 2" <- w630
            n318 = feedback-in #30(w630) -> ()
            n319 = feedback #31(i16 0) -> (w637:i16)
            n320 = Subtract(x=w637, y=w636) -> (x-y=w635:i16)
            "GI Relative phase 2" <- w635
            n321 = feedback-in #31(w635) -> ()
            n322 = And(x=w614, y=w613) -> (x .and. y?=w615:bool)
            n323 = And(x=w615, y="Green FB On/Off") -> (x .and. y?=w645:bool)
            "green FB running" <- w645
            n324 = And(x=w610, y="Red FB On/Off") -> (x .and. y?=w625:bool)
            n325 = Not(x=w608) -> (.not. x?=w607:bool)
            n326 = case shown="True" w625 {
              tunnel: "RI Current Out" -> [w668 _]
              tunnel: [w668 w677] -> w621
              frame False {
              }
              frame True {
                n327 = local read "Red FB Intensity"() -> (w673:i16)
                n328 = Bundle("P4"="P4", "I4"="I4", "D4"="D4") -> (w669:cluster{"P4":i16, "I4":i16, "D4":i16})  [unwired: 1 in]
                n329 = call "Slower PID.vi"("process variable"=w673, "reset?"="Red FB Reset", "setpoint"="Red FB Setpoint", "PID gains (x 2^8)"=w669, "output range"=cluster{"output high":i16, "output low":i16} {"output high"=32767, "output low"=-32768} ("Green FB output range")) -> ("output"=w680:i16)  [unwired: 10 out]
                n330 = To Long Integer(number=w680) -> (32bit integer=w674:i32)
                n331 = Add(x=w674, y=32768) -> (x+y=w676:i32)
                n332 = To Unsigned Word Integer(number=w676) -> (unsigned 16bit integer=w677:u16)
              }
            }
            n333 = And(x=w645, y=w607) -> (x .and. y?=w609:bool)
            n334 = case shown="True" w609 {
              tunnel: "Current Out" -> [w682 w683]
              tunnel: [w682 w683] -> w649
              frame False {
              }
              frame True {
                n335 = disable-structure shown="Disabled" {
                  frame Disabled {
                    n336 = local read "Green FB Sum"() -> (w688:i16)
                    n337 = Bundle("P3"="P3", "I3"="I3", "D3"="D3") -> (w684:cluster{"P3":i16, "I3":i16, "D3":i16})  [unwired: 1 in]
                    n338 = call "Slower PID.vi"("process variable"=w688, "reset?"="Green FB Reset", "setpoint"="Green FB Setpoint", "PID gains (x 2^8)"=w684, "output range"=cluster{"output high":i16, "output low":i16} {"output high"=32767, "output low"=-32768} ("Green FB output range")) -> ("output"=w694:i16)  [unwired: 10 out]
                    n339 = To Long Integer(number=w694) -> (32bit integer=w689:i32)
                    n340 = Add(x=w689, y=32768) -> (x+y=w691:i32)
                    n341 = To Unsigned Word Integer(number=w691) -> ()  [unwired: 1 out]
                  }
                  frame Enabled {
                  }
                }
              }
            }
            n342 = Boolean To (0,1)(Boolean=w610) -> (0, 1=w620:i16)
            n343 = To Unsigned Word Integer(number=w620) -> (unsigned 16bit integer=w622:u16)
            n344 = Boolean To (0,1)(Boolean=w615) -> (0, 1=w651:i16)
            n345 = To Unsigned Word Integer(number=w651) -> (unsigned 16bit integer=w648:u16)
            n346 = Compound Arithmetic op=MULTIPLY(w622, w621) -> (w619:u16)
            n347 = Compound Arithmetic op=MULTIPLY(w648, w649) -> (w650:u16)
          }
        }
      }
      n348 = while "Blue fluorescent laser interlacing (AO control direct to laser)." {
        shift-right: [w521] -> _
        shift-left: w513 -> [w524]
        shift-right: [w518] -> _
        shift-left: i16 0 -> [w516]
        stop <- FALSE stop-if-true
        n349 = flat-sequence {
          tunnel: w524 -> [w527]
          tunnel: [w528] -> w523
          tunnel: [w527] -> w522
          tunnel: [w526] -> w517
          tunnel: w516 -> [w526]
          tunnel: [w531] -> w520
          tunnel: w523 -> [w531]
          tunnel: [w530] -> w519
          tunnel: w522 -> [w530]
          tunnel: w517 -> [w529]
          tunnel: [w541] -> w521
          tunnel: [w557] -> w518
          tunnel: w520 -> [w569]
          tunnel: w519 -> [w566]
          frame #0 {
            n350 = call "Loop Timer13"("Count(Ticks)"=w527) -> ("Tick Count(Ticks)"=w528:u16)
          }
          frame #1 {
            n351 = xnode "FPGA I/O Node"("Connector0/AO3"=w529) -> ()  [unwired: 1 in, 1 out]
          }
          frame #2 {
            n352 = Subtract(x="Blue OFF count (AO)", y="Blue current ON count adj (AO)") -> (x-y=w550:u16)
            n353 = feedback-in #32(w569) -> ()
            n354 = feedback #32(w569) -> (w568:u16)
            n355 = Add(x="Blue current ON count adj (AO)", y="Blue ON count (AO)") -> (x+y=w551:u16)
            n356 = Subtract(x=w569, y=w568) -> (x-y=w567:u16)
            n357 = Subtract(x=w567, y=w566) -> (x-y=w534:u16)
            n358 = Number To Boolean Array(number=w534) -> (Boolean array=w535:bool[])
            n359 = Boolean To (0,1)(Boolean="+ phase (BI AO)") -> (0, 1=w547:i16)
            n360 = Or Array Elements(Boolean array=w535) -> (logical OR=w533:bool)
            n361 = Boolean To (0,1)(Boolean=w533) -> (0, 1=w540:i16)
            n362 = Multiply(x=w547, y="Phase count adjustment (BI AO)") -> (x*y=w543:i16)
            n363 = To Unsigned Byte Integer(number=w540) -> (unsigned 8bit integer=w536:u8)
            n364 = feedback #33(u8 0) -> (w538:u8)
            n365 = Add(x=w536, y=w538) -> (x+y=w537:u8)
            "BI Late Counter (AO)" <- w537
            n366 = feedback-in #33(w537) -> ()
            n367 = feedback #34(i16 0) -> (w544:i16)
            n368 = Subtract(x=w544, y=w543) -> (x-y=w542:i16)
            "BI Relative phase (AO)" <- w542
            n369 = feedback-in #34(w542) -> ()
            n370 = feedback #35(TRUE) -> (w561:bool)
            n371 = case shown="2" "BI Operating Mode (AO)" {
              tunnel: [TRUE FALSE w585] -> w552
              tunnel: w561 -> [_ _ w582]
              frame 0, Default {
              }
              frame 1 {
              }
              frame 2 {
                n372 = Not(x=w582) -> (.not. x?=w584:bool)
                n373 = Select(t=w584, s="Invert BI (AO)", f=w582) -> (s? t:f=w585:bool)
              }
            }
            n374 = And(x=w552, y="Blue FB On/Off") -> (x .and. y?=w553:bool)
            n375 = case shown="True" w553 {
              tunnel: "BI Current Out" -> [w570 _]
              tunnel: [w570 w572] -> w556
              frame False {
              }
              frame True {
                n376 = local read "Blue Intensity"() -> (w571:i16)
                n377 = Bundle("P5"="P5", "I5"="I5", "D5"="D5") -> (w573:cluster{"P5":i16, "I5":i16, "D5":i16})  [unwired: 1 in]
                n378 = call "Slower PID.vi"("process variable"=w571, "reset?"="Blue FB Reset", "setpoint"="Blue FB Setpoint", "PID gains (x 2^8)"=w573, "output range"=cluster{"output high":i16, "output low":i16} {"output high"=32767, "output low"=0} ("Green FB output range")) -> ("output"=w572:i16)  [unwired: 10 out]
              }
            }
            n379 = Not(x=w561) -> (.not. x?=w558:bool)
            n380 = Select(t=w551, s=w558, f=w550) -> (s? t:f=w563:u16)
            n381 = Subtract(x=w563, y=w534) -> (x-y=w545:u16)
            n382 = Add(x=w545, y=w543) -> (x+y=w541:u16)
            n383 = feedback-in #35(w558) -> ()
            n384 = Boolean To (0,1)(Boolean=w552) -> (0, 1=w532:i16)
            n385 = Multiply(x=w532, y=w556) -> (x*y=w557:i16)
          }
        }
      }
    }
    frame Enabled {
    }
  }
  n386 = while "DAQ AI set 1" {
    shift-right: [w702] -> _
    shift-left: w5 -> [w707]
    stop <- FALSE stop-if-true
    n387 = flat-sequence {
      tunnel: w707 -> [w717]
      tunnel: [w718] -> w705
      tunnel: [w717] -> w704
      tunnel: [w728] -> w715
      tunnel: [w727] -> w714
      tunnel: [w726] -> w713
      tunnel: [w725] -> w712
      tunnel: [w724] -> w711
      tunnel: [w723] -> w710
      tunnel: [w722] -> w709
      tunnel: [w721] -> w708
      tunnel: [w720] -> w706
      tunnel: w705 -> [w720]
      tunnel: w704 -> [w719]
      tunnel: [w719] -> w703
      tunnel: [w760] -> w702
      tunnel: w715 -> [w786]
      tunnel: w714 -> [w752]
      tunnel: w713 -> [w753]
      tunnel: w712 -> [w732]
      tunnel: w711 -> [w776]
      tunnel: w710 -> [w775]
      tunnel: w709 -> [w774]
      tunnel: w708 -> [w773]
      tunnel: w706 -> [w770]
      tunnel: w703 -> [w767]
      frame #0 {
        n388 = call "Loop Timer3"("Count(Ticks)"=w717) -> ("Tick Count(Ticks)"=w718:u16)
      }
      frame #1 {
        n389 = xnode "FPGA I/O Node"("Connector1/DIO31"=TRUE ("Connector1/DIO33")) -> ("Connector0/AI0"=w728:i16, "Connector0/AI1"=w727:i16, "Connector0/AI2"=w726:i16, "Connector0/AI3"=w725:i16, "Connector0/AI4"=w724:i16, "Connector0/AI5"=w723:i16, "Connector0/AI6"=w722:i16, "Connector0/AI7"=w721:i16)  [unwired: 9 in, 9 out]
      }
      frame #2 {
        w756 = FALSE ("AI to FIFO")
        # "Normalize by trap bead QPD sum, AI3"
        # "Adjust phase after data acquired if button pressed"
        n390 = feedback #36(i16 1) -> (w779:i16)
        n391 = Increment(x=w779) -> (x+1=w785:i16)
        n392 = Scale By Power Of 2(n="AI1 X Scale", x=w752) -> (x*2^n=w750:i16)
        n393 = Greater?(x=w785, y="N of AI1 Int Acq Sets") -> (0:w782:bool)
        n394 = Select(t=i16 1, s=w782, f=w785) -> (s? t:f=w784:i16)
        n395 = feedback-in #36(w784) -> ()
        n396 = Divide(x=w750, y=w732) -> (x/y=w749:fxp<+/-,16,1>)
        n397 = feedback #37(w756) -> (w754:bool)
        n398 = feedback #38(w756) -> (w772:bool)
        n399 = case shown="1, Default" w779 {
          tunnel: w753 -> [w811 w818 _]
          tunnel: ["Set 1" "Set 2" "Set 3"] -> w777
          tunnel: ["AI to FIFO" w820 w825] -> w771
          tunnel: w772 -> [_ w820 w825]
          tunnel: ["Trap Pos to FIFO" w819 w824] -> w755
          tunnel: w754 -> [_ w819 w824]
          tunnel: w749 -> [w810 w817 _]
          tunnel: [w809 w815 FALSE] -> w736
          tunnel: [w808 w816 u64 0 ("BD1 Frequency Out 2")] -> w735
          frame 1, Default {
            n400 = local read "BD1 Frequency Out 1"() -> (w808:u64)
            n401 = Compound Arithmetic op=AND("Trap Pos to FIFO", "Set 1", "AI to FIFO") -> (w809:bool)
            "AI2 Y Sum Set 1" <- w811
            "AI1 X Set 1" <- w810
          }
          frame 2 {
            n402 = local read "BD1 Frequency Out 2"() -> (w816:u64)
            n403 = Compound Arithmetic op=AND(w819, "Set 2", w820) -> (w815:bool)
            "AI2 Y Sum Set 2" <- w818
            "AI1 X Set 2" <- w817
          }
          frame 3 {
          }
        }
        n404 = And(x=w777, y=w771) -> (x .and. y?=w778:bool)
        n405 = case shown="True" w778 {
          tunnel: w786 -> [_ w839]
          tunnel: w752 -> [_ w838]
          tunnel: w753 -> [_ w837]
          tunnel: w732 -> [_ w836]
          tunnel: w776 -> [_ w835]
          tunnel: w775 -> [_ w834]
          tunnel: w774 -> [_ w833]
          tunnel: w773 -> [_ w832]
          tunnel: 0 ("DMA buffer timeout") -> [_ w841]
          frame False {
          }
          frame True {
            n406 = Build Array(w839, w838, w837, w836, w835, w834, w833, w832) -> (w840:i16[])
            n407 = for {
              tunnel: w840 -> [w843] mode=indexing
              tunnel: w841 -> [w844]
              tunnel: [w842] -> w830 mode=indexing
              n408 = xnode ("FIFO Write")("Element"=w843, "Timeout"=w844) -> ("Timed Out?"=w842:bool)  [unwired: 1 in, 1 out]
            }
            n409 = Or Array Elements(Boolean array=w830) -> (logical OR=w827:bool)
            n410 = Boolean To (0,1)(Boolean=w827) -> (0, 1=w829:i16)
            n411 = feedback #39(u16 0) -> (w828:u16)
            n412 = Add(x=w829, y=w828) -> (x+y=w826:u16)
            "Trap AI FIFO Timeout" <- w826
            n413 = feedback-in #39(w826) -> ()
          }
        }
        n414 = feedback-in #37(w755) -> ()
        n415 = feedback-in #38(w771) -> ()
        n416 = local read "Piezo X out"() -> (w731:i16)
        n417 = local read "Piezo Y out"() -> (w730:i16)
        n418 = case shown="True" w736 {
          tunnel: w735 -> [_ w794]
          tunnel: [u8 0 w791] -> w734
          tunnel: w731 -> [_ w790]
          tunnel: w730 -> [_ w789]
          frame False {
          }
          frame True {
            n419 = Split Number(x=w794) -> (hi(x)=w795:u32, lo(x)=w796:u32)
            n420 = Split Number(x=w795) -> (lo(x)=w797:u16)  [unwired: 1 out]
            n421 = Split Number(x=w796) -> (hi(x)=w798:u16, lo(x)=w799:u16)
            n422 = Build Array "BD 1 nu Stack"(w797, w798, w799, w790, w789) -> (w793:u16[])
            n423 = for {
              tunnel: w793 -> [w806] mode=indexing
              shift-right: [w802] -> w791
              shift-left: u8 0 -> [w803]
              n424 = xnode ("FIFO Method Node")("Element"=w806, "Timeout"="Trap FIFO Set Timeout") -> ("Timed Out?"=w805:bool)  [unwired: 1 in, 1 out]
              n425 = Boolean To (0,1)(Boolean=w805) -> (0, 1=w804:i16)
              n426 = To Unsigned Byte Integer(number=w804) -> (unsigned 8bit integer=w801:u8)
              n427 = Add(x=w801, y=w803) -> (x+y=w802:u8)
            }
          }
        }
        n428 = To Unsigned Word Integer(number=w734) -> (unsigned 16bit integer=w733:u16)
        n429 = feedback #40(u16 0) -> (w747:u16)
        n430 = Add(x=w733, y=w747) -> (x+y=w746:u16)
        "Trap Pos FIFO Timeout" <- w746
        n431 = feedback-in #40(w746) -> ()
        n432 = feedback-in #41(w770) -> ()
        n433 = feedback #41(w770) -> (w769:u16)
        n434 = Subtract(x=w770, y=w769) -> (x-y=w768:u16)
        n435 = xnode "FPGA I/O Node"("Connector1/DIO31"=FALSE ("Connector1/DIO34")) -> ()  [unwired: 1 in, 1 out]
        n436 = Subtract(x=w768, y=w767) -> (x-y=w738:u16)
        n437 = Boolean To (0,1)(Boolean="+ phase") -> (0, 1=w763:i16)
        n438 = Multiply(x=w763, y="Phase count adjustment") -> (x*y=w757:i16)
        n439 = Subtract(x="ai count", y=w738) -> (x-y=w761:u16)
        n440 = Number To Boolean Array(number=w738) -> (Boolean array=w739:bool[])
        n441 = feedback #42(i16 0) -> (w759:i16)
        n442 = Add(x=w761, y=w757) -> (x+y=w760:u16)
        n443 = Subtract(x=w759, y=w757) -> (x-y=w758:i16)
        "Relative phase" <- w758
        n444 = feedback-in #42(w758) -> ()
        n445 = Or Array Elements(Boolean array=w739) -> (logical OR=w737:bool)
        n446 = Boolean To (0,1)(Boolean=w737) -> (0, 1=w744:i16)
        n447 = To Unsigned Byte Integer(number=w744) -> (unsigned 8bit integer=w741:u8)
        n448 = feedback #43(u8 0) -> (w742:u8)
        n449 = Add(x=w741, y=w742) -> (x+y=w740:u8)
        "AI Late Counter" <- w740
        n450 = feedback-in #43(w740) -> ()
      }
    }
  }
  n451 = while "MCL stage control" {
    shift-right: [w868] -> _
    shift-left: w5 -> [w871]
    shift-right: [w861] -> _
    shift-left: w11 -> [w858]
    shift-right: [w860] -> _
    shift-left: w10 -> [w856]
    shift-right: [w855] -> _
    shift-left: w2 -> [w850]
    shift-right: [w853] -> _
    shift-left: w2 -> [w845]
    shift-right: [w851] -> _
    shift-left: w2 -> [w847]
    stop <- FALSE stop-if-true
    n452 = flat-sequence {
      tunnel: w871 -> [w878]
      tunnel: [w879] -> w867
      tunnel: [w878] -> w865
      tunnel: [w877] -> w859
      tunnel: w858 -> [w877]
      tunnel: [w876] -> w857
      tunnel: w856 -> [w876]
      tunnel: w850 -> [w875]
      tunnel: [w875] -> w849
      tunnel: [w874] -> w848
      tunnel: w847 -> [w874]
      tunnel: [w873] -> w846
      tunnel: w845 -> [w873]
      tunnel: w867 -> [w886]
      tunnel: [w886] -> w866
      tunnel: w865 -> [w885]
      tunnel: [w885] -> w864
      tunnel: w859 -> [w884]
      tunnel: w857 -> [w883]
      tunnel: w849 -> [w882]
      tunnel: w848 -> [w881]
      tunnel: w846 -> [w880]
      tunnel: w866 -> [w900]
      tunnel: w864 -> [w899]
      tunnel: [w900] -> w870
      tunnel: [w899] -> w869
      tunnel: [w898] -> w863
      tunnel: [w897] -> w862
      tunnel: [w889] -> w854
      tunnel: [w887] -> w852
      tunnel: [w1007] -> w868
      tunnel: w870 -> [w1014]
      tunnel: w869 -> [w1011]
      tunnel: w863 -> [w1009]
      tunnel: w862 -> [w1008]
      tunnel: [w1009] -> w861
      tunnel: [w1008] -> w860
      tunnel: [w990] -> w855
      tunnel: w854 -> [w990]
      tunnel: [w989] -> w853
      tunnel: w852 -> [w989]
      tunnel: ["Piezo Trap ON/Off (AO3)"] -> w851
      frame #0 {
        n453 = call "Loop Timer5"("Count(Ticks)"=w878) -> ("Tick Count(Ticks)"=w879:u32)
      }
      frame #1 {
        n454 = xnode "FPGA I/O Node"("Connector0/AO1"=w884, "Connector0/AO2"=w883, "Connector0/AO3"=w881, "Connector0/AO4"=w882, "Connector0/AO5"=w880) -> ()  [unwired: 5 in, 5 out]
      }
      frame #2 {
        n455 = local read "Scanning MCL"() -> (w912:bool)
        n456 = Or(x=w912, y="Start scan (MCL)") -> (x .or. y?=w907:bool)
        n457 = Not(x="Abort scan (MCL)") -> (.not. x?=w905:bool)
        n458 = And(x=w905, y=w907) -> (x .and. y?=w904:bool)
        n459 = case "Raster scan" shown="False" w904 {
          tunnel: [w945 w988] -> w909
          tunnel: "Start scan (MCL)" -> [_ w973]
          tunnel: [w945 w949] -> w893
          frame False {
            w945 = i16 0
            n460 = local write "Scanning MCL"(FALSE ("scanning")) -> ()
          }
          frame True {
            w959 = i16 0
            w958 = u64 0
            # "scan incr."
            # "freq. incr. mult."
            # "count steps"
            # "count number of cycles"
            n461 = feedback #44(w958) -> (w985:u64)
            n462 = Select(t=w958, s=w973, f=w985) -> (s? t:f=w987:u64)
            n463 = Increment(x=w987) -> (x+1=w984:u64)
            n464 = Greater?(x="Cycles per step (MCL)", y=w984) -> (0:w968:bool)
            n465 = Select(t=w984, s=w968, f=w958) -> (s? t:f=w983:u64)
            n466 = feedback-in #44(w983) -> ()
            n467 = feedback #45(w958) -> (w982:u64)
            n468 = Select(t=w958, s=w973, f=w982) -> (s? t:f=w977:u64)
            n469 = Increment(x=w977) -> (x+1=w981:u64)
            n470 = Add(x="Scan steps (MCL)", y="Scan steps (MCL)") -> (x+y=w980:u64)
            n471 = Select(t=w977, s=w968, f=w981) -> (s? t:f=w963:u64)
            n472 = Greater?(x=w980, y=w963) -> (0:w962:bool)
            n473 = Select(t=w963, s=w962, f=w958) -> (s? t:f=w978:u64)
            n474 = feedback-in #45(w978) -> ()
            n475 = Equal?(x="Scan steps (MCL)", y=w963) -> (x = y?=w967:bool)
            n476 = Greater?(x="Scan steps (MCL)", y=w977) -> (0:w976:bool)
            n477 = feedback #46(w959) -> (w979:i16)
            n478 = Select(t=w959, s=w973, f=w979) -> (s? t:f=w965:i16)
            n479 = Increment(x=w965) -> (x+1=w975:i16)
            n480 = Decrement(x=w965) -> (x-1=w974:i16)
            n481 = Select(t=w975, s=w976, f=w974) -> (s? t:f=w966:i16)
            n482 = Select(t=w965, s=w967, f=w966) -> (s? t:f=w964:i16)
            n483 = Select(t=w965, s=w968, f=w964) -> (s? t:f=w960:i16)
            n484 = Select(t=w960, s=w962, f=w959) -> (s? t:f=w961:i16)
            n485 = feedback-in #46(w961) -> ()
            n486 = feedback #47(w958) -> (w972:u64)
            n487 = Select(t=w958, s=w973, f=w972) -> (s? t:f=w947:u64)
            n488 = Increment(x=w947) -> (x+1=w969:u64)
            n489 = Select(t=w947, s=w962, f=w969) -> (s? t:f=w948:u64)
            n490 = Greater?(x="Number of scans (MCL)", y=w948) -> (0:w955:bool)
            n491 = Multiply(x="Scan freq.  increment (MCL)", y=w965) -> (x*y=w988:i16)
            n492 = Select(t=TRUE, s="Cont. Scan (MCL)", f=w955) -> (s? t:f=w954:bool)
            "Scanning MCL" <- w954
            n493 = Select(t=w948, s=w954, f=w958) -> (s? t:f=w970:u64)
            n494 = feedback-in #47(w970) -> ()
            n495 = Increment(x=w948) -> (x+1=→"Scan I (MCL)":u64)
            n496 = To Word Integer(number=w947) -> (16bit integer=w950:i16)
            n497 = Multiply(x=w950, y="Scan freq.  increment (MCL)") -> (x*y=w949:i16)
          }
        }
        n498 = case shown="True" "Multiple trap 3 position offset \nfile" {
          tunnel: ["Piezo Trap Y (AO4)" w932] -> w890
          tunnel: ["Piezo Trap X (AO5)" w931] -> w888
          frame False {
          }
          frame True {
            n499 = local read "Scan I"() -> (w943:u64)
            n500 = Decrement(x=w943) -> (x-1=w944:u64)
            n501 = Quotient & Remainder(x=w944, y="Piezo offset Y points") -> (x-y*floor(x/y)=w941:u64, floor(x/y)=w939:u64)
            n502 = Multiply(x=w941, y="Piezo Offset Increment") -> (x*y=w938:u64)
            n503 = Multiply(x="Piezo Offset Increment", y=w939) -> (x*y=w936:u64)
            n504 = Add(x=w936, y="Piezo offset Xmin") -> (x+y=w933:u64)
            n505 = Add(x=w938, y="Piezo Offset Ymin") -> (x+y=w934:u64)
            n506 = To Word Integer(number=w933) -> (16bit integer=w931:i16)
            n507 = To Word Integer(number=w934) -> (16bit integer=w932:i16)
          }
        }
        n508 = Select(t=w893, s="1D or 2D Scan?", f=i16 0) -> (s? t:f=w894:i16)
        n509 = Select(t=w909, s="MCL Scan Axis", f=w894) -> (s? t:f=w910:i16)
        n510 = Select(t=w894, s="MCL Scan Axis", f=w909) -> (s? t:f=w908:i16)
        n511 = case shown="True" "ScanTrap 3 or Fl-laser" {
          tunnel: w910 -> [w920 w922]
          tunnel: w908 -> [w915 w926]
          tunnel: "AO2 (X)" -> [w916 w927]
          tunnel: "AO1 (Y)" -> [w919 w928]
          tunnel: [w918 w928] -> w898
          tunnel: [w917 w927] -> w897
          tunnel: w890 -> [w914 w923]
          tunnel: [w914 w921] -> w889
          tunnel: w888 -> [w913 w925]
          tunnel: [w913 w924] -> w887
          frame False {
            n512 = Add(x=w916, y=w915) -> (x+y=w917:i16)
            n513 = Add(x=w919, y=w920) -> (x+y=w918:i16)
          }
          frame True {
            n514 = Add(x=w923, y=w922) -> (x+y=w921:i16)
            n515 = Add(x=w925, y=w926) -> (x+y=w924:i16)
          }
        }
      }
      frame #3 {
        n516 = feedback-in #48(w1014) -> ()
        n517 = feedback #48(w1014) -> (w1013:u32)
        n518 = Boolean To (0,1)(Boolean="+ phase (MCL)") -> (0, 1=w1005:i16)
        n519 = Subtract(x=w1014, y=w1013) -> (x-y=w1012:u32)
        n520 = Multiply(x=w1005, y="Phase count adjustment (MCL)") -> (x*y=w1001:i16)
        n521 = Subtract(x=w1012, y=w1011) -> (x-y=w993:u32)
        n522 = Subtract(x="MCL count", y=w993) -> (x-y=w1003:u32)
        n523 = feedback #49(i16 0) -> (w1002:i16)
        n524 = Subtract(x=w1002, y=w1001) -> (x-y=w1000:i16)
        "MCL Relative Phase" <- w1000
        n525 = feedback-in #49(w1000) -> ()
        n526 = Number To Boolean Array(number=w993) -> (Boolean array=w994:bool[])
        n527 = Or Array Elements(Boolean array=w994) -> (logical OR=w992:bool)
        n528 = Boolean To (0,1)(Boolean=w992) -> (0, 1=w999:i16)
        n529 = Add(x=w1003, y=w1001) -> (x+y=w1007:u32)
        n530 = To Unsigned Byte Integer(number=w999) -> (unsigned 8bit integer=w996:u8)
        n531 = feedback #50(u8 0) -> (w997:u8)
        n532 = Add(x=w996, y=w997) -> (x+y=w995:u8)
        "MCL Late Counter" <- w995
        n533 = feedback-in #50(w995) -> ()
        "Piezo Y out" <- w990
        "Piezo X out" <- w989
      }
    }
  }
  n534 = while "Trap RF control, main calculations (raster scanning, intensity and position feedback, phase control etc) with primary timing trigger" {
    shift-right: [w1030] -> _
    shift-left: w5 -> [w1029]
    shift-right: [w1028] -> _
    shift-left: FALSE ("Swap F1 and F2") -> [w1027]
    shift-right: [w1023] -> _
    shift-left: u16 0 ("BD 1 Amplitude 3") -> [w1020]
    shift-right: [w1022] -> _
    shift-left: u16 0 ("BD 2 Amplitude 3") -> [w1018]
    shift-right: [w1017] -> _
    shift-left: u64 0 -> [w1016]
    stop <- FALSE stop-if-true
    n535 = flat-sequence {
      tunnel: w1027 -> [w1036]
      tunnel: w1029 -> [w1034]
      tunnel: [w1036] -> w1026
      tunnel: [w1035] -> w1025
      tunnel: [w1034] -> w1024
      tunnel: [w1033] -> w1021
      tunnel: w1020 -> [w1033]
      tunnel: [w1032] -> w1019
      tunnel: w1018 -> [w1032]
      tunnel: [w1047] -> w1030
      tunnel: [w1046] -> w1028
      tunnel: w1026 -> [w1045]
      tunnel: w1025 -> [w1044]
      tunnel: w1024 -> [w1043]
      tunnel: [w1042] -> w1023
      tunnel: [w1041] -> w1022
      tunnel: w1021 -> [w1040]
      tunnel: w1019 -> [w1039]
      tunnel: [w1038] -> w1017
      tunnel: w1016 -> [w1037]
      frame #0 {
        n536 = call "Loop Timer"("Count(Ticks)"=w1034) -> ("Tick Count(Ticks)"=w1035:u16)
      }
      frame #1 {
        n537 = flat-sequence {
          tunnel: w1045 -> [w1055]
          tunnel: w1040 -> [w1049]
          tunnel: w1039 -> [w1048]
          tunnel: [w1117] -> w1047
          tunnel: [w1129] -> w1046
          tunnel: w1044 -> [w1123]
          tunnel: w1043 -> [w1120]
          tunnel: [w1066] -> w1042
          tunnel: [w1065] -> w1041
          tunnel: [w1057] -> w1038
          tunnel: w1037 -> [w1056]
          frame #0 {
            w1050 = -1 ("Timeout")
            # "Operation when you need a long delay for either X or Y to synchonize AOD light out phase (> ~100 ticks)\nor want shorter trap ON timing. Puts some of the delay timing in parallel with the later computations."
            # "Trigger the external loop by sending the boolean FSK value through a FIFO.\nTiming is precise."
            n538 = Boolean To (0,1)(Boolean=w1055) -> (0, 1=w1054:i16)
            n539 = To Unsigned Word Integer(number=w1054) -> (unsigned 16bit integer=w1053:u16)
            n540 = xnode ("FIFO Method Node")("Element"=w1053, "Timeout"=w1050) -> ("FIFO Out"=w1052:refnum<k21>)  [unwired: 1 in, 1 out]
            n541 = xnode ("FIFO Method Node")("Element"=w1049, "Timeout"=w1050, "FIFO In"=w1052) -> ("FIFO Out"=w1051:refnum<k21>)  [unwired: 1 out]
            n542 = xnode ("FIFO Method Node")("Element"=w1048, "Timeout"=w1050, "FIFO In"=w1051) -> ()  [unwired: 2 out]
          }
          frame #1 {
            # "Just counts, wraps around, 8 bit"
            # "Which trap cycle"
            # "Only save the 3rd set's amp in the loop"
            # "If this is NOT set 3 AND NOT (RF synth controls green AND green FB running)\nthen use this sets amp value (otherwise keep the green feedback value)"
            # "Just flips back and forth."
            # "If interlacing is off, this is which cycle to use."
            # "Keep track of trap cycles (trap 1, 2, 3...)"
            # "This is the prior cycle's on time"
            # "increment timing\nindex, reset to 0 if \nend of matrix"
            # "Reset to begginning (1) when number of cycles reached."
            # "timing index"
            # "build byte stacks for writing data\n(must correspond to addresses array constant)"
            # "Timing housekeeping"
            # "Adjust phase if late\n(maintains constant phase relationship between cycles)"
            n543 = feedback #51(u8 0 ("t")) -> (w1126:u8)
            n544 = Increment(x=w1126) -> (x+1=w1165:u8)
            n545 = Increment(x="Number Interlace Cycles") -> (x+1=w1160:u8)
            n546 = Equal?(x=w1165, y=w1160) -> (x = y?=w1167:bool)
            n547 = Select(t=u8 1, s=w1167, f=w1165) -> (s? t:f=w1125:u8)
            n548 = feedback-in #51(w1125) -> ()
            n549 = Increment(x=w1125) -> (x+1=w1162:u8)
            n550 = Equal?(x=w1162, y=w1160) -> (x = y?=w1163:bool)
            n551 = Select "This cycle"(t=u8 1, s=w1163, f=w1162) -> (s? t:f=w1159:u8)
            n552 = Select(t=w1159, s="Interlace ON/OFF", f="Interlace Off Parameters") -> (s? t:f=w1076:u8)
            n553 = feedback-in #52(w1123) -> ()
            n554 = feedback #52(w1123) -> (w1122:u16)
            n555 = Select(t=w1125, s="Interlace ON/OFF", f="Interlace Off Parameters") -> (s? t:f=w1158:u8)
            n556 = Subtract(x=w1123, y=w1122) -> (x-y=w1121:u16)
            n557 = Subtract "The error"(x=w1121, y=w1120) -> (x-y=w1104:u16)
            n558 = case shown="1, Default" w1158 {
              tunnel: ["DIO count 1 (ticks)" "DIO count 2 (ticks)" "DIO count 3 (ticks)"] -> w1119
              frame 1, Default {
              }
              frame 2 {
              }
              frame 3 {
              }
            }
            n559 = Number To Boolean Array(number=w1104) -> (Boolean array=w1105:bool[])
            n560 = Or Array Elements(Boolean array=w1105) -> (logical OR=w1103:bool)
            n561 = Boolean To (0,1)(Boolean=w1103) -> (0, 1=w1110:i16)
            n562 = To Unsigned Byte Integer(number=w1110) -> (unsigned 8bit integer=w1107:u8)
            n563 = feedback #53(u8 0) -> (w1108:u8)
            n564 = Add(x=w1107, y=w1108) -> (x+y=w1106:u8)
            "DIO Late Counter" <- w1106
            n565 = feedback-in #53(w1106) -> ()
            n566 = Subtract(x=w1119, y=w1104) -> (x-y=w1118:u16)
            n567 = local read "green FB running"() -> (w1089:bool)
            n568 = And(x=w1089, y="RF synth bd controls green") -> (x .and. y?=w1088:bool)
            n569 = feedback #54(i64 0 ("y")) -> (w1101:i64)
            n570 = case "Synchronize trap oscillations - always begin/end with trap 1" shown="1, Default" w1076 {
              tunnel: [w1273 w1274 w1275] -> w1102
              tunnel: w1101 -> [w1273 w1274 _]
              frame 2 {
              }
              frame 3 {
              }
              frame 1, Default {
                n571 = Or(x="Osc traps", y="Initiate trap osc") -> (x .or. y?=w1277:bool)
                n572 = case "Trap sine oscillation (or whatever pattern is stored in memory)" shown="True" w1277 {
                  tunnel: [i64 0 ("y") w1281] -> w1275
                  tunnel: "Initiate trap osc" -> [_ w1284]
                  frame False {
                  }
                  frame True {
                    w1288 = u16 0
                    w1286 = -1
                    n573 = local write "Initiate trap osc"(FALSE ("Initiate trap osc")) -> ()
                    n574 = feedback #55(w1288) -> (w1290:u16)
                    n575 = Select(t=w1288, s=w1284, f=w1290) -> (s? t:f=w1289:u16)
                    n576 = Greater Or Equal?(x=w1289, y="Trap osc period (pts)") -> (x >= y?=w1295:bool)
                    n577 = Or(x=w1284, y=w1295) -> (x .or. y?=w1296:bool)
                    n578 = Select(t=u16 0, s=w1296, f=w1289) -> (s? t:f=w1280:u16)
                    n579 = feedback #56(w1286) -> (w1287:i32)
                    n580 = Select(t=w1286, s=w1284, f=w1287) -> (s? t:f=w1285:i32)
                    n581 = Increment(x=w1285) -> (x+1=w1292:i32)
                    n582 = Equal?(x=w1280, y=u16 0) -> (x = y?=w1293:bool)
                    n583 = Increment(x=w1280) -> (x+1=w1300:u16)
                    n584 = feedback-in #55(w1300) -> ()
                    n585 = Select(t=w1292, s=w1293, f=w1285) -> (s? t:f=w1291:i32)
                    n586 = feedback-in #56(w1291) -> ()
                    n587 = case shown="False" "Osc trap cont." {
                      tunnel: w1291 -> [w1304 _]
                      frame False {
                        n588 = Greater Or Equal?(x=w1304, y="N trap osc periods") -> (x >= y?=w1302:bool)
                        n589 = Not(x=w1302) -> (.not. x?=w1301:bool)
                        n590 = local write "Osc traps"(w1301) -> ()
                      }
                      frame True {
                      }
                    }
                    n591 = xnode ("Memory Read")("Address"=w1280, "Memory In"=refnum<k21> "Trap osc memory") -> ("Data"=w1281:i64)  [unwired: 1 out]
                  }
                }
              }
            }
            n592 = case shown="1, Default" w1076 {
              tunnel: [w1318 w1533 "BD 1 Frequency 3"] -> w1155
              tunnel: [w1368 w1532 w1558] -> w1092
              tunnel: ["BD 2 Amplitude 1" "BD 2 Amplitude 2" w1557] -> w1084
              tunnel: [w1315 w1529 "BD 1 Amplitude 3"] -> w1066
              tunnel: "FB Gains" -> [w1338 w1539 _]
              tunnel: "FB output range" -> [w1339 w1538 _]
              tunnel: w1102 -> [w1336 w1536 _]
              tunnel: "BD 2 Frequency 1" -> [w1333 _ _]
              tunnel: "BD 2 Frequency 2" -> [_ w1532 _]
              tunnel: "BD 2 Frequency 3" -> [_ _ w1558]
              tunnel: w1088 -> [_ _ w1556]
              tunnel: [w1318 w1530 w1551] -> w1057
              tunnel: w1056 -> [w1317 w1530 w1551]
              frame 1, Default {
                w1353 = fxp<+/-,24,9> 0.0 ("AI1 X Set 2")
                w1347 = u16 0
                w1365 = u64 0 ("f")
                # "Changed by Ronen - correction \nby PID is now implemented not on \nthe Base BD1 frequency but on the last\nfrequency sent."
                # "Added by Ronen -\nUpper and Lower \nLimits for the FB \ngenerated frequency\nto avoid losing bead \nwhen tether breaks"
                # "Explanation of raster scanning:\n1. Cycles: increment counter by 1 every time interlace cycle returns to trap 1. As long as \n  Cycle per Step is larger than counter, keep incrementing counter and do not change step counter.\n  Once counter is equal to Cycles per step, zero counter and increment step counter.\n2. Steps: Increments up every time cycles counter equals cycles per step. Performs the following:\n- To determine DIRECTION of frequency change:  If ScanstepX2 is EQUAL to step counter (full for-back scan finished)\n   frequency increment is set to zero, AND step counter is set to zero. \n   Otherwise: if no change to step counter (because cycleperstep>cycle counter), then no change to frequency\n   increment. \n   If step counter has changed (cycleperstep=cycle counter), then need to figure out direction of frequency change:\n   if step counter is EQUAL to Scansteps: No change to frequency increment\n   Otherwise: If scan steps > step counter - 1 (forward scan NOT completed): increment frequency by 1\n                       If scan steps equal or smaller than step counter -1 (forward scan completed): increment frequency by -1\n\n3. Scans: Increment scan counter every time step counter equals 2Xscan steps (full for-back scan completed)\n    if number of scans > scan counter: Send TRUE to scanning, continue scan\n    if number of scans = scan counter: Send FALSE to Scanning, Scan finished.\n\n  The wire with the asterik can be used as the index for getting the mirror positions in the offset scan."
                # "This signal integration happens no matter what\nso that correct setpoints can be chosen before \nturning on the FB."
                # "Trap 1"
                n593 = local read "AI1 X Set 2"() -> (w1330:fxp<+/-,16,1>)
                n594 = local read "AI1 X Set 1"() -> (w1350:fxp<+/-,16,1>)
                n595 = local read "Scanning"() -> (w1369:bool)
                n596 = Multiply(x=w1330, y="B factor") -> (x*y=w1328:fxp<+/-,48,17>)
                n597 = Or(x=w1369, y="Start scan") -> (x .or. y?=w1363:bool)
                n598 = case shown="True" "Diff FB Measurement?" {
                  tunnel: w1328 -> [w1386 w1395]
                  tunnel: w1350 -> [w1385 w1396]
                  tunnel: [w1383 w1387] -> w1351
                  frame False {
                    n599 = Select(t=w1385, s="Trap Pos FB Monitor T1 or T2", f=w1386) -> (s? t:f=w1383:fxp<+/-,48,17>)
                  }
                  frame True {
                    n600 = Subtract(x=w1396, y=w1395) -> (x-y=w1388:fxp<+/-,48,17>)
                    n601 = Not(x="Negate Diff?") -> (.not. x?=w1394:bool)
                    n602 = Boolean To (0,1)(Boolean="Negate Diff?") -> (0, 1=w1392:i16)
                    n603 = Boolean To (0,1)(Boolean=w1394) -> (0, 1=w1393:i16)
                    n604 = Negate(x=w1392) -> (-x=w1391:i16)
                    n605 = Add(x=w1391, y=w1393) -> (x+y=w1389:i16)
                    n606 = Multiply(x=w1389, y=w1388) -> (x*y=w1387:fxp<+/-,63,32>)
                  }
                }
                n607 = Not(x="Abort scan") -> (.not. x?=w1361:bool)
                n608 = And(x=w1361, y=w1363) -> (x .and. y?=w1360:bool)
                n609 = case "For raster scanning" shown="True" w1360 {
                  tunnel: [u64 0 w1519] -> w1366
                  tunnel: "Start scan" -> [_ w1504]
                  tunnel: [u64 1 w1481] -> w1331
                  frame False {
                    n610 = local write "Scanning"(FALSE ("scanning")) -> ()
                  }
                  frame True {
                    w1488 = i64 0
                    w1487 = u64 0
                    # "scan incr."
                    # "freq. incr. mult."
                    # "count steps"
                    # "count number of cycles"
                    n611 = feedback #57(w1487) -> (w1516:u64)
                    n612 = Select(t=w1487, s=w1504, f=w1516) -> (s? t:f=w1518:u64)
                    n613 = Increment(x=w1518) -> (x+1=w1515:u64)
                    n614 = Greater?(x="Cycles per step", y=w1515) -> (0:w1497:bool)
                    n615 = Select(t=w1515, s=w1497, f=w1487) -> (s? t:f=w1514:u64)
                    n616 = feedback-in #57(w1514) -> ()
                    n617 = feedback #58(w1487) -> (w1513:u64)
                    n618 = Select(t=w1487, s=w1504, f=w1513) -> (s? t:f=w1508:u64)
                    n619 = Increment(x=w1508) -> (x+1=w1512:u64)
                    n620 = Add(x="Scan steps", y="Scan steps") -> (x+y=w1511:u64)
                    n621 = Select(t=w1508, s=w1497, f=w1512) -> (s? t:f=w1492:u64)
                    n622 = Greater?(x=w1511, y=w1492) -> (0:w1491:bool)
                    n623 = Select(t=w1492, s=w1491, f=w1487) -> (s? t:f=w1509:u64)
                    n624 = feedback-in #58(w1509) -> ()
                    n625 = Equal?(x="Scan steps", y=w1492) -> (x = y?=w1496:bool)
                    n626 = Greater?(x="Scan steps", y=w1508) -> (0:w1507:bool)
                    n627 = feedback #59(w1488) -> (w1510:i64)
                    n628 = Select(t=w1488, s=w1504, f=w1510) -> (s? t:f=w1494:i64)
                    n629 = Increment(x=w1494) -> (x+1=w1506:i64)
                    n630 = Decrement(x=w1494) -> (x-1=w1505:i64)
                    n631 = Select(t=w1506, s=w1507, f=w1505) -> (s? t:f=w1495:i64)
                    n632 = Select(t=w1494, s=w1496, f=w1495) -> (s? t:f=w1493:i64)
                    n633 = Select(t=w1494, s=w1497, f=w1493) -> (s? t:f=w1489:i64)
                    n634 = Select(t=w1489, s=w1491, f=w1488) -> (s? t:f=w1490:i64)
                    n635 = feedback-in #59(w1490) -> ()
                    n636 = feedback #60(w1487) -> (w1503:u64)
                    n637 = Select(t=w1487, s=w1504, f=w1503) -> (s? t:f=w1499:u64)
                    n638 = Increment(x=w1499) -> (x+1=w1500:u64)
                    n639 = Select(t=w1499, s=w1491, f=w1500) -> (s? t:f=w1498:u64)
                    n640 = Greater?(x="Number of scans", y=w1498) -> (0:w1484:bool)
                    n641 = Multiply(x="Scan freq.  increment", y=w1494) -> (x*y=w1519:i64)
                    n642 = Select(t=TRUE, s="Cont. Scan", f=w1484) -> (s? t:f=w1483:bool)
                    "Scanning" <- w1483
                    n643 = Select(t=w1498, s=w1483, f=w1487) -> (s? t:f=w1501:u64)
                    n644 = feedback-in #60(w1501) -> ()
                    n645 = Increment(x=w1498) -> (x+1=w1481:u64)
                  }
                }
                "Scan I" <- w1331
                n646 = feedback #61(w1347) -> (w1346:u16)
                n647 = Increment(x=w1346) -> (x+1=w1348:u16)
                n648 = Greater Or Equal?(x=w1348, y="Trap Pos FB Int Count") -> (x >= y?=w1316:bool)
                n649 = Select(t=w1347, s=w1316, f=w1348) -> (s? t:f=w1349:u16)
                n650 = feedback-in #61(w1349) -> ()
                n651 = feedback #62(w1353) -> (w1352:fxp<+/-,24,9>)
                n652 = Add(x=w1351, y=w1352) -> (x+y=w1345:fxp<+/-,24,9>)
                n653 = case "Trap 1 X intensity feedback" shown="True" "FB On/Off Set 1" {
                  tunnel: "BD 1 Amplitude 1" -> [w1521 _]
                  tunnel: [w1521 w1525] -> w1315
                  tunnel: w1339 -> [_ w1522]
                  tunnel: w1338 -> [_ w1523]
                  frame False {
                  }
                  frame True {
                    n654 = local read "AI2 Y Sum Set 1"() -> (w1526:i16)
                    n655 = call "Slower PID.vi"("process variable"=w1526, "reset?"="FB Reset Set 1", "setpoint"="FB Setpoint Set 1", "PID gains (x 2^8)"=w1523, "output range"=w1522) -> ("output"=w1527:i16)  [unwired: 10 out]
                    n656 = To Unsigned Word Integer(number=w1527) -> (unsigned 16bit integer=w1525:u16)
                  }
                }
                "BD1 amplitude 1 out" <- w1315
                n657 = Select(t=w1353, s=w1316, f=w1345) -> (s? t:f=w1356:fxp<+/-,24,9>)
                n658 = feedback-in #62(w1356) -> ()
                n659 = Divide(x=w1345, y="Trap Pos FB Int Count") -> (x/y=w1340:fxp<+/-,16,1>)
                n660 = feedback #63(fxp<+/-,24,9> 0.0 ("AI1 X Set 2")) -> (w1357:fxp<+/-,24,9>)
                n661 = Select(t=w1345, s=w1316, f=w1357) -> (s? t:f=w1358:fxp<+/-,24,9>)
                "Trap Pos FB Int Signal" <- w1358
                n662 = feedback-in #63(w1358) -> ()
                n663 = feedback #64(fxp<+/-,16,1> 0.0 ("Trap Pos FB Int-Norm Signal")) -> (w1342:fxp<+/-,16,1>)
                n664 = Select(t=w1340, s=w1316, f=w1342) -> (s? t:f=w1341:fxp<+/-,16,1>)
                "Trap Pos FB Int-Norm Signal" <- w1341
                n665 = feedback-in #64(w1341) -> ()
                n666 = case "For position feedback" shown="True" "Force feedback" {
                  tunnel: [i64 0 w1402] -> w1323
                  tunnel: w1340 -> [_ w1399]
                  tunnel: w1316 -> [_ w1398]
                  frame False {
                  }
                  frame True {
                    n667 = feedback #65(i64 0) -> (w1401:i64)
                    n668 = case shown="False" w1398 {
                      tunnel: [w1403 w1407] -> w1402
                      tunnel: w1401 -> [w1403 _]
                      tunnel: w1399 -> [_ w1406]
                      frame False {
                      }
                      frame True {
                        n669 = xnode ("PID")("process variable"=w1406, "reset?"="Trap Pos. FB Reset", "setpoint"="Trap Pos. FB SP", "PID gains"="Trap Pos. FB Gains", "output range"="Trap pos. FB Range") -> ("output"=w1416:fxp<+/-,16,1>)
                        n670 = Negate(x=w1416) -> (-x=w1415:fxp<+/-,17,2>)
                        n671 = Select(t=w1415, s="Trap Pos FB Negate Action", f=w1416) -> (s? t:f=w1412:fxp<+/-,17,2>)
                        n672 = Scale By Power Of 2(n=u32 15, x=u32 1) -> (x*2^n=w1409:u32)
                        n673 = Multiply(x=w1412, y=w1409) -> (x*y=w1408:fxp<+/-,17,17>)
                        n674 = To Quad Integer(1:w1408) -> (0:w1420:i64)
                        "Trap Pos FB Action" <- w1420
                        n675 = Multiply(x=w1420, y="Trap Pos. FB Mult Factor") -> (x*y=w1418:i64)
                        n676 = Add(x=w1418, y="Trap Pos. FB Offset Factor") -> (x+y=w1407:i64)
                        n677 = disable-structure shown="Disabled" {
                          disable-tunnel: w1407 -> [w1427 _]
                          frame Disabled {
                            w1431 = u32 0
                            n678 = feedback #66() -> (w1428:i64)  [unwired: 1 in]
                            n679 = Add(x=w1427, y=w1428) -> (x+y=w1425:i64)
                            n680 = feedback #67(w1431) -> (w1433:u32)
                            n681 = Increment(x=w1433) -> (x+1=w1422:u32)
                            n682 = Greater Or Equal?(x=w1422, y="FB Trig Integrate") -> (x >= y?=w1423:bool)
                            n683 = Select(t=i64 0, s=w1423, f=w1425) -> (s? t:f=w1429:i64)
                            n684 = feedback-in #66(w1429) -> ()
                            n685 = Select(t=w1431, s=w1423, f=w1422) -> (s? t:f=w1432:u32)
                            n686 = feedback-in #67(w1432) -> ()
                            n687 = And(x=w1423, y="FPGA Trap Trig") -> (x .and. y?=w1430:bool)
                            n688 = case "Trap FB trigger excitation laser ON" shown="True" w1430 {
                              tunnel: w1425 -> [_ w1437]
                              tunnel: w1422 -> [_ w1435]
                              frame False {
                              }
                              frame True {
                                n689 = Not(x="TTrig Negate Pos") -> (.not. x?=w1444:bool)
                                n690 = Boolean To (0,1)(Boolean="TTrig Negate Pos") -> (0, 1=w1442:i16)
                                n691 = Boolean To (0,1)(Boolean=w1444) -> (0, 1=w1443:i16)
                                n692 = Negate(x=w1442) -> (-x=w1441:i16)
                                n693 = Add(x=w1441, y=w1443) -> (x+y=w1440:i16)
                                n694 = Multiply(x=w1440, y=w1437) -> (x*y=w1439:i64)
                                "TTrig Sig" <- w1439
                                n695 = Multiply(x="FPGA TTrig Thresh", y=w1435) -> (x*y=w1436:i64)
                                "TTrig Fin Thresh" <- w1436
                                n696 = Greater Or Equal?(x=w1439, y=w1436) -> (x >= y?=w1438:bool)
                                n697 = case shown="True" w1438 {
                                frame False {
                                }
                                frame True {
                                w1447 = TRUE ("Green FB On/Off")
                                w1449 = u8 2 ("Operating Mode")
                                n698 = local write "Operating Mode 2"(w1449) -> ()
                                n699 = local write "Operating Mode"(w1449) -> ()
                                n700 = local write "Green FB On/Off"(w1447) -> ()
                                n701 = local write "FPGA Trap Trig"(FALSE ("FPGA Trap Trig")) -> ()
                                "TTrig?" <- w1447
                                }
                                }
                              }
                            }
                          }
                          frame Enabled {
                          }
                        }
                      }
                    }
                    n702 = feedback-in #65(w1402) -> ()
                  }
                }
                n703 = And(x="Force feedback", y="Dynamic Force FB (Ronen)") -> (x .and. y?=w1325:bool)
                n704 = case shown="True" w1325 {
                  tunnel: w1323 -> [w1374 w1378]
                  tunnel: [w1373 w1377] -> w1324
                  tunnel: w1317 -> [_ w1376]
                  tunnel: w1316 -> [_ w1375]
                  frame False {
                    # "(BD1 Frequency 1)"
                    n705 = Add(x="BD 1 Frequency 1", y=w1374) -> (x+y=w1373:u64)
                  }
                  frame True {
                    n706 = case shown="True" w1375 {
                      tunnel: w1378 -> [_ w1382]
                      tunnel: [w1379 w1381] -> w1377
                      tunnel: w1376 -> [w1379 w1380]
                      frame False {
                      }
                      frame True {
                        n707 = Add(x=w1380, y=w1382) -> (x+y=w1381:u64)
                      }
                    }
                  }
                }
                n708 = Select(t=w1336, s="Trap 1 osc enable", f=i64 0) -> (s? t:f=w1334:i64)
                n709 = Select(t=w1365, s="Scan BD", f=w1366) -> (s? t:f=w1364:u64)
                n710 = Select(t=w1366, s="Scan BD", f=w1365) -> (s? t:f=w1322:u64)
                n711 = Add(x=w1364, y=w1333) -> (x+y=w1368:u64)
                n712 = Compound Arithmetic op=ADD(w1334, w1324, w1322) -> (w1321:u64)
                n713 = In Range and Coerce(upper limit="FB Max Frequency", x=w1321, lower limit="FB Min frequency") -> (coerced(x)=w1318:u64)  [unwired: 1 out]
                "BD1 Frequency Out 1" <- w1318
              }
              frame 2 {
                # "Trap 2"
                n714 = case "Trap 2 X intensity feedback" shown="True" "FB On/Off Set 2" {
                  tunnel: [w1543 w1546] -> w1529
                  tunnel: "BD 1 Amplitude 2" -> [w1543 _]
                  tunnel: w1539 -> [_ w1545]
                  tunnel: w1538 -> [_ w1544]
                  frame False {
                  }
                  frame True {
                    n715 = local read "AI2 Y Sum Set 2"() -> (w1549:i16)
                    n716 = call "Slower PID.vi"("process variable"=w1549, "reset?"="FB Reset Set 2", "setpoint"="FB Setpoint Set 2", "PID gains (x 2^8)"=w1545, "output range"=w1544) -> ("output"=w1547:i16)  [unwired: 10 out]
                    n717 = To Unsigned Word Integer(number=w1547) -> (unsigned 16bit integer=w1546:u16)
                  }
                }
                "BD1 amplitude 2 out" <- w1529
                n718 = Select(t=w1536, s="Trap 2 osc enable", f=i64 0) -> (s? t:f=w1535:i64)
                n719 = Add(x="BD 1 Frequency 2", y=w1535) -> (x+y=w1533:u64)
                "BD1 Frequency Out 2" <- w1533
              }
              frame 3 {
                # "Remember if FB was previously on/off"
                # "Fluorescence period"
                n720 = feedback #68(FALSE) -> (w1552:bool)
                n721 = case shown="True" w1556 {
                  tunnel: [w1562 w1578] -> w1557
                  tunnel: "BD 2 Amplitude 3" -> [w1562 _]
                  tunnel: [FALSE TRUE] -> w1553
                  tunnel: w1552 -> [_ w1563]
                  frame False {
                  }
                  frame True {
                    # "Makes it so first time FB run when turned on, the PID sees the detector intensity from the last time FB was running, rather than something near zero. Especially assuming the setpoint is not changing, this will make the FB more stable when resuming, and not overshoot the turnon intensity."
                    # "FB output range: 0 should be low, full scale is 12 bits.\nBut be careful not to go over, then higher bits just get ignored by RF board, so output will actually jump down and be unstable. Keep it under 4000 to be safe."
                    n722 = local read "Green FB Sum"() -> (w1566:i16)
                    n723 = feedback-in #69(w1566) -> ()
                    n724 = feedback #69(i16 0 ("Green FB Sum")) -> (w1565:i16)
                    n725 = Select(t=w1566, s=w1563, f=w1565) -> (s? t:f=w1564:i16)
                    n726 = Bundle("P3 2"="P3 2", "I3 2"="I3 2", "D3 2"="D3 2") -> (w1577:cluster{"P3 2":i16, "I3 2":i16, "D3 2":i16})  [unwired: 1 in]
                    n727 = Bundle("RF synth green feedback max"="RF synth green feedback max", i16 0) -> (w1569:cluster{"RF synth green feedback max":i16, i16})  [unwired: 1 in]
                    n728 = call "Slower PID.vi"("process variable"=w1564, "reset?"="Green FB Reset 2", "setpoint"="Green FB Setpoint 2", "PID gains (x 2^8)"=w1577, "output range"=w1569) -> ("output"=w1579:i16)  [unwired: 10 out]
                    n729 = To Unsigned Word Integer(number=w1579) -> (unsigned 16bit integer=w1578:u16)
                  }
                }
                n730 = feedback-in #68(w1553) -> ()
              }
            }
            n731 = feedback-in #54(w1102) -> ()
            n732 = Split Number(x=w1155) -> (hi(x)=w1154:u32, lo(x)=w1153:u32)
            n733 = Boolean To (0,1)(Boolean="+ phase (DIO)") -> (0, 1=w1115:i16)
            n734 = Split Number(x=w1154) -> (lo(x)=w1152:u16)  [unwired: 1 out]
            n735 = Split Number(x=w1153) -> (hi(x)=w1151:u16, lo(x)=w1150:u16)
            n736 = Split Number(x=w1152) -> (hi(x)=w1144:u8, lo(x)=w1143:u8)
            n737 = Split Number(x=w1151) -> (hi(x)=w1142:u8, lo(x)=w1141:u8)
            n738 = Split Number(x=w1150) -> (hi(x)=w1140:u8, lo(x)=w1139:u8)
            n739 = Multiply(x=w1115, y="Phase count adjustment (DIO)") -> (x*y=w1111:i16)
            n740 = feedback #70(TRUE) -> (w1098:bool)
            n741 = Not(x=w1098) -> (.not. x?=w1097:bool)
            n742 = feedback-in #70(w1097) -> ()
            n743 = feedback #71(i16 0) -> (w1113:i16)
            n744 = Subtract(x=w1113, y=w1111) -> (x-y=w1112:i16)
            "DIO Relative phase" <- w1112
            n745 = feedback-in #71(w1112) -> ()
            n746 = Add(x=w1118, y=w1111) -> (x+y=w1117:u16)
            n747 = Build Array "BD 1 nu Stack"(w1144, w1143, w1142, w1141, w1140, w1139) -> (w1138:u8[])
            n748 = Not Equal?(x=w1076, y=u8 3) -> (x != y?=w1085:bool)
            n749 = case "Store in RF board F1 or F2" shown="True" w1097 {
              tunnel: [w1306 w1310] -> w1129
              tunnel: [u8 10 u8 4] -> w1130
              tunnel: "Swap F1 and F2" -> [w1307 w1310]
              tunnel: "BD 2 Frequency 1" -> [_ w1309]
              tunnel: "BD 2 Frequency 2" -> [w1305 _]
              tunnel: [w1305 w1309] -> w1093
              frame False {
                # "for RF synth controls\ngreen: F1/F2 stay same"
                # "F2 address (hex)"
                n750 = Not(x=w1307) -> (.not. x?=w1306:bool)
              }
              frame True {
                # "low chooses F1"
                # "F1 address (hex)"
              }
            }
            n751 = Select(t=w1093, s="RF synth bd controls green", f=w1092) -> (s? t:f=w1091:u64)
            n752 = Split Number(x=w1091) -> (hi(x)=w1149:u32, lo(x)=w1148:u32)
            n753 = Split Number(x=w1149) -> (lo(x)=w1147:u16)  [unwired: 1 out]
            n754 = Split Number(x=w1148) -> (hi(x)=w1146:u16, lo(x)=w1145:u16)
            n755 = Split Number(x=w1147) -> (hi(x)=w1137:u8, lo(x)=w1136:u8)
            n756 = Split Number(x=w1146) -> (hi(x)=w1135:u8, lo(x)=w1134:u8)
            n757 = Split Number(x=w1145) -> (hi(x)=w1133:u8, lo(x)=w1132:u8)
            n758 = feedback #72(u16 0 ("BD 2 Amplitude 3")) -> (w1082:u16)
            n759 = Select(t=w1082, s=w1085, f=w1084) -> (s? t:f=w1083:u16)
            n760 = feedback-in #72(w1083) -> ()
            n761 = And(x=w1085, y=w1088) -> (x .and. y?=w1087:bool)
            n762 = Build Array "BD 2 nu Stack"(w1137, w1136, w1135, w1134, w1133, w1132) -> (w1131:u8[])
            n763 = Select(t=w1082, s=w1087, f=w1084) -> (s? t:f=w1065:u16)
            n764 = flat-sequence "Update trap RF synth board settings to be used for the upcoming trap cycle." {
              tunnel: w1131 -> [w1222]
              tunnel: w1138 -> [w1223]
              tunnel: [w1223] -> w1080
              tunnel: [w1222] -> w1079
              tunnel: w1130 -> [w1224]
              tunnel: w1080 -> [w1226]
              tunnel: w1079 -> [w1225]
              tunnel: w1067 -> [w1237]
              tunnel: w1069 -> [w1236]
              tunnel: w1068 -> [w1235]
              frame #0 {
                # "To possibly delay\nthese writes to very\nend of loop (for x and\ny phase adjust)"
                n765 = call "Wait8"("Count(Ticks)"="Next trap write delay (ticks)") -> ()  [unwired: 1 out]
              }
              frame #1 {
                # "Next trap RF frequency:\n\nWrite next trap cycle frequency to buffer."
                n766 = for {
                  tunnel: w1226 -> [w1232] mode=indexing
                  tunnel: w1225 -> [w1231] mode=indexing
                  tunnel: w1224 -> [w1229]
                  i -> [w1230]
                  n767 = To Unsigned Byte Integer(number=w1230) -> (unsigned 8bit integer=w1227:u8)
                  n768 = Add(x=w1229, y=w1227) -> (x+y=w1228:u8)
                  n769 = call "write to RF synth bd.vi"("Address Byte"=w1228, "BD 2 Byte"=w1231, "BD 1 Byte"=w1232) -> ()
                }
              }
              frame #2 {
                w1233 = TRUE ("Connector1/DIO15")
                # "Send udclk high\n(BD 1 and 2) to make the new frequency active in F1 or F2 word. But it won't actually be the used frequency until FSK switches to it (begining of next cycle)."
                n770 = xnode "FPGA I/O Node"("Connector1/DIO30"=w1233, "Connector1/DIO29"=w1233) -> ()  [unwired: 2 in, 2 out]
              }
              frame #3 {
                w1234 = FALSE ("Connector1/DIO15")
                n771 = xnode "FPGA I/O Node"("Connector1/DIO30"=w1234, "Connector1/DIO29"=w1234) -> ()  [unwired: 2 in, 2 out]
              }
              frame #4 {
                # "Next trap RF phase offset:\n\nSet the next trap cycle amplitude to the buffer. Won't become active until udclk is set high at proper time at the begining of the next cycle."
                n772 = case shown="True" w1237 {
                  tunnel: w1236 -> [_ w1238]
                  tunnel: w1235 -> [_ w1239]
                  frame False {
                  }
                  frame True {
                    # "phase 1 address start"
                    n773 = for {
                      tunnel: w1238 -> [w1246] mode=indexing
                      tunnel: w1239 -> [w1245] mode=indexing
                      tunnel: u8 0 -> [w1243]
                      i -> [w1244]
                      n774 = To Unsigned Byte Integer(number=w1244) -> (unsigned 8bit integer=w1241:u8)
                      n775 = Add(x=w1243, y=w1241) -> (x+y=w1242:u8)
                      n776 = call "write to RF synth bd.vi"("Address Byte"=w1242, "BD 2 Byte"=w1245, "BD 1 Byte"=w1246) -> ()
                    }
                  }
                }
              }
              frame #5 {
                # "Prep to reset RF phase to zero at start of next cycle. Only reset BD 1. Do nothing to BD 2. This puts the settings in the buffer. A udclk high will make both this phase reset and possibly a new phase offset setting active."
                n777 = case shown="True" "RF phase reset before cycles" {
                  frame False {
                  }
                  frame True {
                    w1249 = u8 66  # BD 1 reset
                    n778 = call "write to RF synth bd.vi"("Address Byte"=u8 31, "BD 2 Byte"=u8 2, "BD 1 Byte"=w1249) -> ()
                  }
                }
              }
              frame #6 {
                # "Address"
                # "Data BD 2"
                # "Data BD 1"
                # "If phase reset wasn't chosen previously, these actions will have no affect. For both BD's, data should be binary 10, and address should be hex 1F (bin 01 1111)"
                # "This sets up the digital communication lines to restart phase accumulation (start RF running agin). It cancels out the possible phase reset. Just need to set WR DIO low then udclk DIOhigh  to make this happen. Doing this here early (and not using the usual board write function) speeds things up.\n\nRestarts RF (BD 1 only, BD2 never stopped in first place)."
                n779 = xnode "FPGA I/O Node"("Connector1/DIO0"=FALSE, "Connector1/DIO1"=FALSE, "Connector1/DIO2"=FALSE, "Connector1/DIO3"=FALSE, "Connector1/DIO4"=FALSE, "Connector1/DIO5"=FALSE, "Connector1/DIO6"=TRUE, "Connector1/DIO7"=FALSE, "Connector1/DIO8"=FALSE, "Connector1/DIO9"=TRUE, "Connector1/DIO10"=TRUE, "Connector1/DIO11"=TRUE, "Connector1/DIO12"=TRUE, "Connector1/DIO13"=TRUE, "Connector1/DIO20"=FALSE, "Connector1/DIO21"=FALSE, "Connector1/DIO22"=FALSE, "Connector1/DIO23"=FALSE, "Connector1/DIO24"=FALSE, "Connector1/DIO25"=FALSE, "Connector1/DIO26"=TRUE, "Connector1/DIO27"=FALSE) -> ()  [unwired: 22 in, 22 out]
              }
            }
            n780 = feedback #73(fxp<+,8,8> 0.0) -> (w1062:fxp<+,8,8>)
            n781 = Increment(x=w1062) -> (x+1=w1060:fxp<+,8,8>)
            n782 = feedback-in #73(w1060) -> ()
            n783 = case "Trap RF phase offset control methods" shown="3" "Phase offset method" {
              tunnel: [fxp<+,14,14> 0.0 ("Phase BD 1") w1172 w1187 w1216] -> w1070
              tunnel: "Phase Trap 1" -> [_ w1173 w1188 _]
              tunnel: w1076 -> [_ w1174 w1189 w1217]
              tunnel: [FALSE TRUE TRUE TRUE] -> w1067
              tunnel: "Phase Trap 2" -> [_ w1170 w1185 _]
              tunnel: w1060 -> [_ _ w1184 _]
              frame 0, Default {
              }
              frame 1 {
                # "Constant increment of phase offset with each trap cycle. This results in a constant phase difference between trap cycles. \nOnly for traps 1 and 2 (set phase offset to zero for set three)."
                n784 = case shown="1, Default" w1174 {
                  tunnel: w1173 -> [_ _ w1180]
                  tunnel: [w1176 fxp<+,14,14> 0.0 w1181] -> w1172
                  tunnel: w1170 -> [w1175 _ _]
                  frame 2 {
                    n785 = feedback #74(fxp<+,14,14> 0.0) -> (w1178:fxp<+,14,14>)
                    n786 = Add(x=w1175, y=w1178) -> (x+y=w1176:fxp<+,14,14>)
                    n787 = feedback-in #74(w1176) -> ()
                  }
                  frame 3 {
                  }
                  frame 1, Default {
                    n788 = feedback #75(fxp<+,14,14> 0.0) -> (w1183:fxp<+,14,14>)
                    n789 = Add(x=w1180, y=w1183) -> (x+y=w1181:fxp<+,14,14>)
                    n790 = feedback-in #75(w1181) -> ()
                  }
                }
              }
              frame 2 {
                # "Changing increment of phase offset with each trap cycle. This results in a constant change in phase difference between trap cycles. \nOnly for traps 1 and 2 (set phase offset to zero for set three)."
                n791 = case shown="2" w1189 {
                  tunnel: w1188 -> [_ _ w1199]
                  tunnel: [w1190 fxp<+,14,14> 0.0 w1197] -> w1187
                  tunnel: w1185 -> [w1192 _ _]
                  tunnel: w1184 -> [w1193 _ w1200]
                  frame 2 {
                    n792 = Multiply(x=w1192, y=w1193) -> (x*y=w1191:fxp<+,16,16>)
                    n793 = feedback #76(fxp<+,14,14> 0.0) -> (w1195:fxp<+,14,14>)
                    n794 = Add(x=w1191, y=w1195) -> (x+y=w1190:fxp<+,14,14>)
                    n795 = feedback-in #76(w1190) -> ()
                  }
                  frame 3 {
                  }
                  frame 1, Default {
                    n796 = Multiply(x=w1199, y=w1200) -> (x*y=w1198:fxp<+,16,16>)
                    n797 = feedback #77(fxp<+,14,14> 0.0) -> (w1202:fxp<+,14,14>)
                    n798 = Add(x=w1198, y=w1202) -> (x+y=w1197:fxp<+,14,14>)
                    n799 = feedback-in #77(w1197) -> ()
                  }
                }
              }
              frame 3 {
                w1209 = u32 1013904223  # LCG constant C (add)
                w1211 = fxp<+,21,21> 1664525.0  # LCG constant A (multiply)
                # "Set a random phase offset. Random number generated using the LCG method. Constants and method taken from NI white noise generator code (method is general though)."
                # "shift to 14 significant bits"
                n800 = feedback #78(u32 4294967295 ("seed")) -> (w1206:u32)
                n801 = Multiply(x=w1206, y=w1211) -> (x*y=w1210:u32)
                n802 = Split Number(x=w1206) -> (hi(x)=w1212:u16)  [unwired: 1 out]
                n803 = To Unsigned Word Integer(number=w1212) -> (unsigned 16bit integer=w1204:u16)
                n804 = Add(x=w1210, y=w1209) -> (x+y=w1208:fxp<+,32,32>)
                n805 = To Unsigned Long Integer(number=w1208) -> (unsigned 32bit integer=w1205:u32)
                n806 = feedback-in #78(w1205) -> ()
                n807 = Scale By Power Of 2(n=i8 -2 ("Uniform scale factor"), x=w1204) -> (x*2^n=w1213:u16)
                n808 = To Fixed-Point(number=w1213) -> (fixed-point=w1203:fxp<+,14,14>)  [unwired: 1 in]
                "Random phase generated" <- w1203
                n809 = case shown="1, Default" w1217 {
                  tunnel: [w1218 fxp<+,14,14> 0.0 w1220] -> w1216
                  tunnel: w1203 -> [w1218 _ w1220]
                  frame 2 {
                  }
                  frame 3 {
                  }
                  frame 1, Default {
                  }
                }
              }
            }
            n810 = To Unsigned Word Integer(number=w1070) -> (unsigned 16bit integer=w1075:u16)
            n811 = Split Number(x=w1075) -> (hi(x)=w1073:u8, lo(x)=w1074:u8)
            n812 = Split Number(x=u16 0) -> (hi(x)=w1071:u8, lo(x)=w1072:u8)
            n813 = Build Array ("BD 1 A Stack")(w1073, w1074) -> (w1069:u8[])
            n814 = Build Array ("BD 1 A Stack")(w1071, w1072) -> (w1068:u8[])
          }
        }
      }
    }
  }
  n815 = while "RF synth board interlacing timing loop" {
    tunnel: w5 -> [_]
    stop <- FALSE stop-if-true
    # "This loop is stalled until the RF FIFO get a value. With this method we gain additional delay time (because  we allow the rest of the main RF loop to procede while this loop waits to send the switch signals - a form of parallelism). This helps to simplify the main RF code. \n\nThe code also allow optimal interlacing while also controlling trap RF phase. \n\nNote: a lot of work has gone into optimizing these methods and it is unclear how they can be made any faster or better than this (many failed tries). Right now there is essentially ~4 ticks (~90 ns ns) of imperfection in the switching from trap 1 to trap 2. ~2 ticks of no RF (phase reset) then ~2 ticks of trap 2 with the wrong amplitude (T1 amplitude). The total ticks is 200, so not a big error.\n\nPhase can be precisely set for each trap. Phase reset and switching, has similar delays as fsk frequency switching. And phase reset and phase offset changes are also not simultaneous. So we can't perfectly line everything up.\n\nIf you start from amp zero though (as for trap 1), the on switch is perfect. Likewise the off is perfect for trap 2. \n\nThe green laser switching is also perfect because of its reduced duty cycle and delays in fsk switching between 80 and 0 MHz."
    n816 = xnode ("FIFO Read")("Timeout"=-1) -> ("Element"=w1626:u16, "FIFO Out"=w1622:refnum<k21>)  [unwired: 1 in, 1 out]
    n817 = Equal To 0?(x=w1626) -> (x = 0?=w1623:bool)
    n818 = Not(x=w1623) -> (.not. x?=w1580:bool)
    n819 = flat-sequence "BD 1 and 2 RF phase and amplitude switching" {
      tunnel: w1580 -> [_]
      tunnel: w1615 -> [w1730]
      tunnel: w1614 -> [w1729]
      tunnel: w1613 -> [w1728]
      tunnel: w1612 -> [w1727]
      tunnel: w1611 -> [w1726]
      tunnel: w1610 -> [w1725]
      tunnel: w1609 -> [w1724]
      tunnel: w1608 -> [w1723]
      tunnel: w1606 -> [w1722]
      tunnel: w1605 -> [w1721]
      tunnel: w1604 -> [w1720]
      tunnel: w1602 -> [w1718]
      tunnel: w1601 -> [w1717]
      tunnel: w1600 -> [w1716]
      tunnel: w1603 -> [w1719]
      tunnel: w1607 -> [w1715]
      tunnel: w1599 -> [w1754]
      tunnel: w1598 -> [w1753]
      tunnel: w1597 -> [w1752]
      tunnel: w1596 -> [w1751]
      tunnel: w1595 -> [w1750]
      tunnel: w1594 -> [w1749]
      tunnel: w1593 -> [w1748]
      tunnel: w1592 -> [w1747]
      tunnel: w1591 -> [w1746]
      tunnel: w1589 -> [w1745]
      tunnel: w1588 -> [w1744]
      tunnel: w1587 -> [w1743]
      tunnel: w1586 -> [w1742]
      tunnel: w1585 -> [w1741]
      tunnel: w1584 -> [w1740]
      tunnel: w1590 -> [w1739]
      frame #0 {
        # "Delay to align amp/frequency switching depending on the method used.\n\nCan also give enough time to do the parallel amplitude calculations"
        n820 = call "Wait"("Count(Ticks)"="Amp switch delay") -> ()  [unwired: 1 out]
      }
      frame #1 {
        w1710 = TRUE ("Connector1/DIO30")
        # "make phase offset and phase reset active with buffer transfer"
        n821 = xnode "FPGA I/O Node"("Connector1/DIO29"=w1710, "Connector1/DIO30"=w1710) -> ()  [unwired: 2 in, 2 out]
      }
      frame #2 {
        w1711 = FALSE ("Connector1/DIO15")
        # "write phase restart to buffer and reset udclk"
        n822 = xnode "FPGA I/O Node"("Connector1/DIO29"=w1711, "Connector1/DIO30"=w1711, "Connector1/DIO15"=FALSE ("Connector1/DIO14")) -> ()  [unwired: 3 in, 3 out]
      }
      frame #3 {
        w1713 = TRUE ("Connector1/DIO15")
        # "make phase restart active"
        # "reset WR"
        n823 = xnode "FPGA I/O Node"("Connector1/DIO15"=w1713, "Connector1/DIO29"=w1713, "Connector1/DIO30"=w1713) -> ()  [unwired: 3 in, 3 out]
      }
      frame #4 {
        w1714 = FALSE ("Connector1/DIO30")
        # "Address"
        # "set amp byte 1, and reset udclk"
        n824 = xnode "FPGA I/O Node"("Connector1/DIO0"=w1730, "Connector1/DIO1"=w1729, "Connector1/DIO2"=w1728, "Connector1/DIO3"=w1727, "Connector1/DIO4"=w1726, "Connector1/DIO5"=w1725, "Connector1/DIO6"=w1724, "Connector1/DIO7"=w1723, "Connector1/DIO8"=TRUE, "Connector1/DIO9"=FALSE, "Connector1/DIO10"=FALSE, "Connector1/DIO11"=FALSE, "Connector1/DIO12"=FALSE, "Connector1/DIO13"=TRUE, "Connector1/DIO20"=w1715, "Connector1/DIO21"=w1722, "Connector1/DIO22"=w1721, "Connector1/DIO23"=w1720, "Connector1/DIO24"=w1719, "Connector1/DIO25"=w1718, "Connector1/DIO26"=w1717, "Connector1/DIO27"=w1716, "Connector1/DIO30"=w1714, "Connector1/DIO29"=w1714) -> ()  [unwired: 24 in, 24 out]
      }
      frame #5 {
        # "write amp byte 1 to buffer"
        n825 = xnode "FPGA I/O Node"("Connector1/DIO15"=FALSE ("Connector1/DIO14")) -> ()  [unwired: 1 in, 1 out]
      }
      frame #6 {
        # "reset WR"
        n826 = xnode "FPGA I/O Node"("Connector1/DIO15"=TRUE) -> ()  [unwired: 1 in, 1 out]
      }
      frame #7 {
        # "Address"
        # "set amp byte 2"
        n827 = xnode "FPGA I/O Node"("Connector1/DIO0"=w1754, "Connector1/DIO1"=w1753, "Connector1/DIO2"=w1752, "Connector1/DIO3"=w1751, "Connector1/DIO4"=w1750, "Connector1/DIO5"=w1749, "Connector1/DIO6"=w1748, "Connector1/DIO7"=w1747, "Connector1/DIO8"=TRUE, "Connector1/DIO9"=FALSE, "Connector1/DIO10"=FALSE, "Connector1/DIO11"=FALSE, "Connector1/DIO12"=TRUE, "Connector1/DIO13"=FALSE, "Connector1/DIO20"=w1746, "Connector1/DIO21"=w1739, "Connector1/DIO22"=w1745, "Connector1/DIO23"=w1744, "Connector1/DIO24"=w1743, "Connector1/DIO25"=w1742, "Connector1/DIO26"=w1741, "Connector1/DIO27"=w1740) -> ()  [unwired: 22 in, 22 out]
      }
      frame #8 {
        # "write amp byte 2"
        n828 = xnode "FPGA I/O Node"("Connector1/DIO15"=FALSE ("Connector1/DIO14")) -> ()  [unwired: 1 in, 1 out]
      }
      frame #9 {
        w1762 = TRUE ("Connector1/DIO15")
        # "transfer amp bytes 1 and 2 and reset WR"
        n829 = xnode "FPGA I/O Node"("Connector1/DIO29"=w1762, "Connector1/DIO30"=w1762, "Connector1/DIO15"=TRUE ("Connector1/DIO14")) -> ()  [unwired: 3 in, 3 out]
      }
      frame #10 {
        w1764 = FALSE ("Connector1/DIO14")
        # "reset udclk"
        n830 = xnode "FPGA I/O Node"("Connector1/DIO29"=w1764, "Connector1/DIO30"=w1764) -> ()  [unwired: 2 in, 2 out]
      }
    }
    n831 = flat-sequence "FSK BD 1 (trap X)" {
      tunnel: w1580 -> [w1628]
      tunnel: [w1628] -> w1583
      tunnel: w1583 -> [w1629]
      frame #0 {
        n832 = call "Wait2"("Count(Ticks)"="BD 1 Delay (ticks)") -> ()  [unwired: 1 out]
      }
      frame #1 {
        # "switch frequency"
        n833 = xnode "FPGA I/O Node"("Connector1/DIO36"=w1629) -> ()  [unwired: 1 in, 1 out]
      }
    }
    n834 = flat-sequence "FSK BD 2 (trap Y or green laser AOM)" {
      tunnel: w1580 -> [w1766]
      tunnel: [w1766] -> w1625
      tunnel: w1625 -> [w1767]
      frame #0 {
        n835 = call "Wait11"("Count(Ticks)"="BD 2 Delay (Ticks)") -> ()  [unwired: 1 out]
      }
      frame #1 {
        # "switch frequency"
        n836 = xnode "FPGA I/O Node"("Connector1/DIO37"=w1767) -> ()  [unwired: 1 in, 1 out]
      }
    }
    n837 = xnode ("FIFO Read")("Timeout"=-1, "FIFO In"=w1622) -> ("Element"=w1617:u16, "FIFO Out"=w1621:refnum<k21>)  [unwired: 1 out]
    n838 = xnode ("FIFO Read")("Timeout"=-1, "FIFO In"=w1621) -> ("Element"=w1616:u16)  [unwired: 2 out]
    n839 = node-c288() -> (w1619:T6)  [unwired: 1 in]
    n840 = timed-loop "Convert amplitude words to bits" {
      timing: w1619 -> [_]
      timing-out: [_] -> w1618
      tunnel: w1617 -> [w1686]
      tunnel: w1616 -> [w1685]
      tunnel: [w1662] -> w1615
      tunnel: [w1661] -> w1614
      tunnel: [w1660] -> w1613
      tunnel: [w1659] -> w1612
      tunnel: [w1658] -> w1611
      tunnel: [w1657] -> w1610
      tunnel: [w1656] -> w1609
      tunnel: [w1655] -> w1608
      tunnel: [w1654] -> w1607
      tunnel: [w1653] -> w1606
      tunnel: [w1652] -> w1605
      tunnel: [w1651] -> w1604
      tunnel: [w1650] -> w1603
      tunnel: [w1649] -> w1602
      tunnel: [w1648] -> w1601
      tunnel: [w1647] -> w1600
      tunnel: [w1646] -> w1599
      tunnel: [w1645] -> w1598
      tunnel: [w1644] -> w1597
      tunnel: [w1643] -> w1596
      tunnel: [w1642] -> w1595
      tunnel: [w1641] -> w1594
      tunnel: [w1640] -> w1593
      tunnel: [w1639] -> w1592
      tunnel: [w1638] -> w1591
      tunnel: [w1637] -> w1590
      tunnel: [w1636] -> w1589
      tunnel: [w1635] -> w1588
      tunnel: [w1634] -> w1587
      tunnel: [w1633] -> w1586
      tunnel: [w1632] -> w1585
      tunnel: [w1631] -> w1584
      stop <- TRUE stop-if-true
      # "Board 1 Data"
      # "Board 2 Data"
      # "Board 1 Data"
      # "Board 2 Data"
      n841 = Split Number(x=w1686) -> (hi(x)=w1684:u8, lo(x)=w1664:u8)
      n842 = Split Number(x=w1685) -> (hi(x)=w1683:u8, lo(x)=w1663:u8)
      n843 = Number To Boolean Array(number=w1684) -> (Boolean array=w1704:bool[])
      n844 = Number To Boolean Array(number=w1683) -> (Boolean array=w1695:bool[])
      n845 = Index Array(array=w1704, index=7) -> (element=w1662:bool)
      n846 = Index Array(array=w1704, index=6) -> (element=w1661:bool)
      n847 = Index Array(array=w1704, index=5) -> (element=w1660:bool)
      n848 = Index Array(array=w1704, index=4) -> (element=w1659:bool)
      n849 = Index Array(array=w1704, index=3) -> (element=w1658:bool)
      n850 = Index Array(array=w1704, index=2) -> (element=w1657:bool)
      n851 = Index Array(array=w1704, index=1) -> (element=w1656:bool)
      n852 = Index Array(array=w1704, index=0) -> (element=w1655:bool)
      n853 = Index Array(array=w1695, index=7) -> (element=w1654:bool)
      n854 = Index Array(array=w1695, index=6) -> (element=w1653:bool)
      n855 = Index Array(array=w1695, index=5) -> (element=w1652:bool)
      n856 = Index Array(array=w1695, index=4) -> (element=w1651:bool)
      n857 = Index Array(array=w1695, index=3) -> (element=w1650:bool)
      n858 = Index Array(array=w1695, index=2) -> (element=w1649:bool)
      n859 = Index Array(array=w1695, index=1) -> (element=w1648:bool)
      n860 = Index Array(array=w1695, index=0) -> (element=w1647:bool)
      n861 = Number To Boolean Array(number=w1664) -> (Boolean array=w1682:bool[])
      n862 = Number To Boolean Array(number=w1663) -> (Boolean array=w1673:bool[])
      n863 = Index Array(array=w1682, index=7) -> (element=w1646:bool)
      n864 = Index Array(array=w1682, index=6) -> (element=w1645:bool)
      n865 = Index Array(array=w1682, index=5) -> (element=w1644:bool)
      n866 = Index Array(array=w1682, index=4) -> (element=w1643:bool)
      n867 = Index Array(array=w1682, index=3) -> (element=w1642:bool)
      n868 = Index Array(array=w1682, index=2) -> (element=w1641:bool)
      n869 = Index Array(array=w1682, index=1) -> (element=w1640:bool)
      n870 = Index Array(array=w1682, index=0) -> (element=w1639:bool)
      n871 = Index Array(array=w1673, index=7) -> (element=w1638:bool)
      n872 = Index Array(array=w1673, index=6) -> (element=w1637:bool)
      n873 = Index Array(array=w1673, index=5) -> (element=w1636:bool)
      n874 = Index Array(array=w1673, index=4) -> (element=w1635:bool)
      n875 = Index Array(array=w1673, index=3) -> (element=w1634:bool)
      n876 = Index Array(array=w1673, index=2) -> (element=w1633:bool)
      n877 = Index Array(array=w1673, index=1) -> (element=w1632:bool)
      n878 = Index Array(array=w1673, index=0) -> (element=w1631:bool)
    }
    n879 = node-c288(w1618) -> ()
  }
  n880 = while "Control APD data integration - stream to host" {
    shift-right: [w1777] -> _
    shift-left: w7 -> [w1782]
    shift-right: [w1773] -> _
    shift-left: w6 -> [w1771]
    shift-right: [w1772] -> _
    shift-left: w6 -> [w1770]
    stop <- FALSE stop-if-true
    # "red laser"
    # "green laser"
    n881 = flat-sequence {
      tunnel: w1782 -> [w1786]
      tunnel: [w1787] -> w1780
      tunnel: [w1786] -> w1778
      tunnel: w1771 -> [w1785]
      tunnel: w1770 -> [w1784]
      tunnel: [w1785] -> w1769
      tunnel: [w1784] -> w1768
      tunnel: [w1799] -> w1781
      tunnel: w1780 -> [w1799]
      tunnel: [w1798] -> w1779
      tunnel: w1778 -> [w1798]
      tunnel: [w1797] -> w1776
      tunnel: [w1796] -> w1775
      tunnel: [w1790] -> w1774
      tunnel: w1769 -> [w1789]
      tunnel: w1768 -> [w1788]
      tunnel: [w1864] -> w1777
      tunnel: w1781 -> [w1873]
      tunnel: w1779 -> [w1870]
      tunnel: w1776 -> [w1857]
      tunnel: w1775 -> [w1856]
      tunnel: w1774 -> [w1844]
      tunnel: [w1832] -> w1773
      tunnel: [w1831] -> w1772
      frame #0 {
        n882 = call "Loop Timer6"("Count(Ticks)"=w1786) -> ("Tick Count(Ticks)"=w1787:u32)
      }
      frame #1 {
        n883 = flat-sequence {
          tunnel: [w1803] -> w1795
          tunnel: w1789 -> [w1801]
          tunnel: w1788 -> [w1800]
          tunnel: w1795 -> [w1806]
          tunnel: [w1810] -> w1794
          tunnel: [w1809] -> w1793
          tunnel: [w1806] -> w1792
          tunnel: [w1805] -> w1791
          tunnel: [w1817] -> w1796
          tunnel: [w1818] -> w1797
          tunnel: w1794 -> [w1818]
          tunnel: w1793 -> [w1817]
          tunnel: w1792 -> [w1816]
          tunnel: w1791 -> [w1815]
          tunnel: [w1815] -> w1790
          frame #0 {
            # "use separate variable so each APD won't\nhave to wait to read"
            n884 = feedback #79(FALSE) -> (w1802:bool)
            "APD1 out state" <- w1802
            "APD2 out state" <- w1802
            "APD3 out state" <- w1802
            n885 = Not(x=w1802) -> (.not. x?=w1803:bool)
            n886 = feedback-in #79(w1803) -> ()
            "ALEX green ON" <- w1801
            "ALEX red ON" <- w1800
          }
          frame #1 {
            n887 = local read "APD 3 Counts 1"() -> (w1808:u32)
            n888 = local read "APD 3 Counts 0"() -> (w1807:u32)
            n889 = local read "APD 1 Counts 1"() -> (w1814:u32)
            n890 = local read "APD 1 Counts 0"() -> (w1813:u32)
            n891 = local read "APD 2 Counts 1"() -> (w1812:u32)
            n892 = local read "APD 2 Counts 0"() -> (w1811:u32)
            n893 = Select(t=w1808, s=w1806, f=w1807) -> (s? t:f=w1805:u32)
            n894 = Select(t=w1814, s=w1806, f=w1813) -> (s? t:f=w1810:u32)
            n895 = Select(t=w1812, s=w1806, f=w1811) -> (s? t:f=w1809:u32)
          }
          frame #2 {
            n896 = case shown="False" w1816 {
              frame False {
                w1819 = u32 0 ("APD 1 Counts 0")
                n897 = local write "APD 1 Counts 0"(w1819) -> ()
                n898 = local write "APD 2 Counts 0"(w1819) -> ()
                n899 = local write "APD 3 Counts 0"(w1819) -> ()
              }
              frame True {
                w1820 = u32 0 ("APD 1 Counts 1")
                n900 = local write "APD 1 Counts 1"(w1820) -> ()
                n901 = local write "APD 2 Counts 1"(w1820) -> ()
                n902 = local write "APD 3 Counts 1"(w1820) -> ()
              }
            }
          }
        }
      }
      frame #2 {
        w1823 = TRUE
        w1826 = i16 1
        # "crude initialization: if APD to FIFO is off (usually\nonly before initializing a measurement) count is forced to 0\nand green to true"
        # "ALEX: switch between green and red laser for a specified # of counts\neach. No blue laser integration yet."
        # "red laser"
        # "green laser"
        # "switch green or red"
        # "count cycles till switching"
        n903 = feedback-in #80(w1873) -> ()
        n904 = feedback #80(w1873) -> (w1872:u32)
        n905 = Subtract(x=w1873, y=w1872) -> (x-y=w1871:u32)
        n906 = Subtract(x=w1871, y=w1870) -> (x-y=w1849:u32)
        n907 = case shown="True" "APD to FIFO" {
          tunnel: w1857 -> [_ w1878]
          tunnel: w1856 -> [_ w1876]
          tunnel: w1844 -> [_ w1874]
          frame False {
          }
          frame True {
            n908 = flat-sequence {
              tunnel: 0 ("Timeout") -> [w1880]
              tunnel: w1878 -> [w1881]
              tunnel: [w1880] -> w1877
              tunnel: w1877 -> [w1882]
              tunnel: w1876 -> [w1883]
              tunnel: [w1882] -> w1875
              tunnel: w1875 -> [w1885]
              tunnel: w1874 -> [w1884]
              frame #0 {
                n909 = xnode ("FIFO Write")("Element"=w1881, "Timeout"=w1880) -> ()  [unwired: 1 in, 2 out]
              }
              frame #1 {
                n910 = xnode ("FIFO Write")("Element"=w1883, "Timeout"=w1882) -> ()  [unwired: 1 in, 2 out]
              }
              frame #2 {
                n911 = xnode ("FIFO Write")("Element"=w1884, "Timeout"=w1885) -> ()  [unwired: 1 in, 2 out]
              }
            }
          }
        }
        n912 = Subtract(x="APD Acq Rate Count", y=w1849) -> (x-y=w1865:u32)
        n913 = Number To Boolean Array(number=w1849) -> (Boolean array=w1850:bool[])
        n914 = Or Array Elements(Boolean array=w1850) -> (logical OR=w1848:bool)
        n915 = Boolean To (0,1)(Boolean=w1848) -> (0, 1=w1855:i16)
        n916 = To Unsigned Byte Integer(number=w1855) -> (unsigned 8bit integer=w1852:u8)
        n917 = feedback #81(u8 0) -> (w1853:u8)
        n918 = Add(x=w1852, y=w1853) -> (x+y=w1851:u8)
        "APD Acq Late Counter" <- w1851
        n919 = feedback-in #81(w1851) -> ()
        n920 = Boolean To (0,1)(Boolean="+ phase (APD Acq)") -> (0, 1=w1861:i16)
        n921 = Multiply(x=w1861, y="Phase Count Adjustment (APD Acq)") -> (x*y=w1858:i16)
        n922 = Add(x=w1865, y=w1858) -> (x+y=w1864:u32)
        n923 = feedback #82(i16 0) -> (w1863:i16)
        n924 = Subtract(x=w1863, y=w1858) -> (x-y=w1860:i16)
        "APD Acq Relative Phase" <- w1860
        n925 = feedback-in #82(w1860) -> ()
        n926 = feedback #83(w1826) -> (w1827:i16)
        n927 = Select(t=w1827, s="APD to FIFO", f=w1826) -> (s? t:f=w1825:i16)
        n928 = Increment(x=w1825) -> (x+1=w1828:i16)
        n929 = To Word Integer(number=w1857) -> (16bit integer=w1866:i16)
        n930 = To Word Integer(number=w1844) -> (16bit integer=w1845:i16)
        n931 = To Word Integer(number=w1856) -> (16bit integer=w1867:i16)
        n932 = Multiply(x="APD AO scale factor", y=w1867) -> (x*y=w1846:i16)
        n933 = Multiply(x="APD AO scale factor", y=w1845) -> (x*y=w1842:i16)
        n934 = Multiply(x="APD AO scale factor", y=w1866) -> (x*y=w1847:i16)
        n935 = feedback #84(w1823) -> (w1822:bool)
        n936 = Select(t=w1822, s="APD to FIFO", f=w1823) -> (s? t:f=w1821:bool)
        n937 = Select(t="ALEX green on count", s=w1821, f="ALEX red on count") -> (s? t:f=w1838:i16)
        n938 = Greater?(x=w1825, y=w1838) -> (0:w1837:bool)
        n939 = Select(t=i16 1, s=w1837, f=w1828) -> (s? t:f=w1835:i16)
        n940 = feedback-in #83(w1835) -> ()
        n941 = Not(x=w1821) -> (.not. x?=w1839:bool)
        n942 = xnode "FPGA I/O Node"("Connector0/AO5"=w1847, "Connector0/AO7"=w1846, "Connector0/AO6"=w1842) -> ()  [unwired: 3 in, 3 out]
        n943 = Select(t=w1839, s=w1837, f=w1821) -> (s? t:f=w1834:bool)
        n944 = feedback-in #84(w1834) -> ()
        n945 = Not(x=w1834) -> (.not. x?=w1833:bool)
        n946 = Not(x="ALEX ON") -> (.not. x?=w1829:bool)
        n947 = Or(x=w1833, y=w1829) -> (x .or. y?=w1831:bool)
        n948 = Or(x=w1829, y=w1834) -> (x .or. y?=w1832:bool)
      }
    }
  }
